vi "多点监测上位机-网络版.vi"() -> ()   [LabVIEW 2017]
uses:
  <vilib>/Utility/miscctls.llb/LVRowAndColumnTypeDef.ctl
  <vilib>/Utility/miscctls.llb/LVRowAndColumnUnsignedTypeDef.ctl
  <vilib>/Platform/TimedLoop/XDataNode/timing_clust.ctl
  <vilib>/Platform/TimedLoop/XDataNode/nitl_modes.ctl
  <vilib>/Platform/TimedLoop/XDataNode/wakeup.ctl
  <vilib>/Instr/_visa.llb/VISA Find Search Mode.ctl
  <vilib>/sound2/lvsound2.llb/Sound File Info (path).vi
  <vilib>/sound2/lvsound2.llb/Sound File Read Open.vi
  <vilib>/sound2/lvsound2.llb/Sound File Read (DBL).vi
  <vilib>/Utility/inputDevices.llb/closeMouse.vi
  <vilib>/Utility/inputDevices.llb/mouseAcquire.vi
  <vilib>/Platform/TimedLoop/XDataNode/XDataNode.xnode
  <vilib>/Platform/TimedLoop/XDataNode/XDNodeRunTimeDep.lvlib
  <vilib>/Utility/xml.llb/Read From XML File(string).vi
panel:
  out "信号-状态栏可见行数":bool=TRUE
  in  "定时器":T1
  in  "标志-定时分段?":bool=TRUE
  in  "菜单锁-报警表":bool=TRUE
  in  "菜单锁-设备表":bool=TRUE
  out "手动静音窗口VI-引用":refnum<vi>
  in  "报警列表提示索引":i32
  in  "设备列表提示索引":i32
  out "监测数量限值":cluster{"min":i32, "max":i32}
  out "监-停止信号":refnum<vi>
  in  "报警列表提示":string[](array[string])=["选行技巧：按住 ctl 可离散选择，按住 shift 可范围选择，ctl+A 选择全部行", "右键菜单：多选后 某些项可批量操作", "双击“单元格”：打开报警记录数据分析界面，可编辑结论、生成Word报表"]
  in  "设备列表提示":string[](array[string])=["选行技巧：按住 ctl 可离散选择，按住 shift 可范围选择，ctl+A 选择全部行", "右键菜单：多选后 某些项可批量操作", "双击“状态”列：启用或禁用设备（某些版本中禁用此功能）", "双击“设备信息”列：修改设备信息", "双击“一级限值”列：修改报警限值", "双击“网络地址”列：删除设备", "双击“空白行”：添加设备"]
  in  "停止信号":enum16{"内部停止信号", "外部停止信号"}(ring)
  out "新纪录通知VI":refnum<vi>
  in  "新记录簇":cluster{"新记录列表行":string[], "对应缓存文件":string}[](array[cluster])
  in  "报警记录数":i32
  in  "蜂鸣音效":waveform(dbl)[](array[waveform]) caption="数据"
  in  "新记录？":bool=TRUE
  in  "Right":i16
  in  "Left":i16
  in  "探头数":i32
  out "定时循环结构名称":string="采集探头属性"
  in  "测量状态":T2
  in  "通信单元-探头属性引用[]":refnum<vi>[](array[refnum])
  out "通信单元-改动项引用[]":refnum<vi>[](array[refnum])
  out "监测窗口VI":refnum<vi>
  out "报警记录缓存数据文件":string[](array[string])
  in  "监测模式":bool caption="方格样式"
  in  "查看报表":bool caption="方格样式"
  in  "设置":bool
  in  "通知设置":bool caption="方格样式"
  out "公司LOGO与型号":bool
  out "设备表名":string="设备列表"
  in  "串口配置":bool
  in  "设备表-修改信息":bool
  in  "设备表-报警设置":bool
  in  "状态栏-项名[]":string[](array[string])
  in  "设备表-累积定时":bool
  in  "设备表-累积清零":bool
  in  "设备表-添加设备":bool
  in  "设备表-删除设备":bool
  in  "设备排序":bool
  in  "设备表-排序":bool
  out "设备列表操作提示":string
  out "定时触发VI-引用":refnum<vi>
  out "通信单元-VI引用[]":refnum<vi>[](array[refnum])
  in  "探头属性数组":T3[](array[typedef])
  in  "菜单项-实时列表":T12=enum."禁用"
  in  "实时数据列表":i32[](listbox)
  out "报警表名":string="报警记录"
  in  "报警表-刷新":bool
  in  "报警表-预览":bool
  in  "报警表-删除":bool
  out "报警列表操作提示":string
  in  "报警表-复制":bool
  in  "菜单项-报警列表":T13=enum."预览并生成报表"
  in  "报警记录列表":i32[](listbox)
  in  "状态类型":enum16{"全部", "报警", "通信", "设置"}(ring)
  in  "暂停更新？":bool
  in  "状态栏":i32(listbox)
  in  "开机启动":bool
  in  "device ID":refnum<k1> caption="设备ID"
  in  "监测模式？":bool
  out "点到行列-实时列表":T14 caption="单元格位置"
  out "点到行列-报警记录":T14 caption="单元格位置"
  out "停止":bool=TRUE
  in  "清除状态":bool
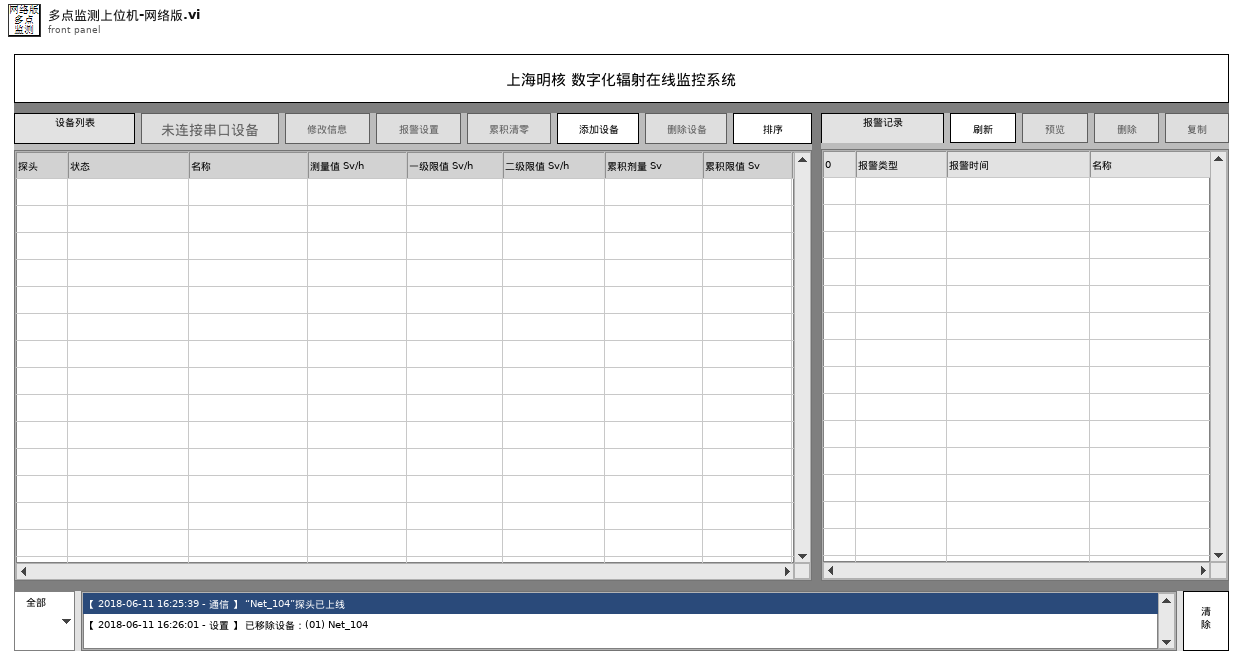
[diagram p1: front panel]
types:
  T1 = typedef "定时器枚举.ctl" = enum16{"累积定时", "导出定时"}
  T2 = typedef "测量状态.ctl" = enum16{"正常", "一级报警", "二级报警", "累积报警", "有掉线"}
  T3 = typedef "探头属性.ctl" = cluster{"探头地址与信息":T4, "测量值":T7, "限值":T8, "探头状态":T9, "累积记录":T10, "报警方式":T11}
  T4 = typedef "探测器信息.ctl" = cluster{"网络地址":string, "名称":string, "备注":string, "累积剂量":dbl, "累积限值":dbl, "硬件剂量率限值":T5, "剂量率限值1":dbl, "剂量率限值2":dbl, "报警方式":T6}
  T5 = typedef "探头剂量率限值选择.ctl" = enum16{"一级限值", "二级限值"}
  T6 = typedef "报警方式选择.ctl" = enum16{"常报警", "自动静音", "手动静音"}
  T7 = typedef "测量值.ctl" = cluster{"时间":timestamp, "数值":dbl}
  T8 = typedef "剂量率限值.ctl" = cluster{"限值1":dbl, "限值2":dbl, "探头限值":T5}
  T9 = typedef "探头状态.ctl" = enum16{"正常", "离线", "禁用", "一级报警", "二级报警", "累积报警"}
  T10 = typedef "单条累积记录.ctl" = cluster{"起始时间":timestamp, "结束时间":timestamp, "累积剂量":dbl}
  T11 = typedef "报警方式.ctl" = cluster{"报警方式":T6, "延迟计时":u16, "报警中？":bool}
  T12 = typedef "菜单项-实时列表.ctl" = enum16{"启用", "禁用", "修改探头信息", "修改报警设置", "设备排序", "重启累积时段", "累积定时", "累积清零", "添加设备", "删除设备"}
  T13 = typedef "菜单项-报警列表.ctl" = enum16{"刷新", "预览并生成报表", "删除记录", "复制选中项至剪贴板"}
  T14 = typedef "LVRowAndColumnTypeDef.ctl" = cluster{"Row":i32, "Column":i32}
  T15 = typedef "LVRowAndColumnUnsignedTypeDef.ctl" = cluster{"Row":u32, "Column":u32}
  T16 = typedef "簇-输入.ctl" = cluster{"配置文件动作":T17, "数据输入":variant}
  T17 = typedef "枚举-配置文件动作.ctl" = enum16{"初始化加载配置", "读取配置", "写入-屏幕键盘", "写入-静音延迟", "写入-主要探头类型", "写入-串口配置", "写入-累积定时", "写入-导出定时", "保存配置到文件"}
  T18 = enum32{"Invalid", "Standard", "Closed", "Hidden", "Minimized", "Maximized"}
  T19 = typedef "XDNodeRunTimeDep.lvlib/timing_clust.ctl" = cluster{"Expected End [f-1]":u64, "Actual End [f-1]":u64, "Finished Late? [f-1]":bool, "Expected End [i-1]":u64, "Actual End [i-1]":u64, "Finished Late? [i-1]":bool, "Expected Start [i]":u64, "Actual Start [i]":u64, "Expected Start [f]":u64, "Actual Start [f]":u64, "Source Name":string, "Structure Name":string, "Period":i64, "Deadline":i64, "Offset":i64, "Start":i64, "Priority":i32, "Timeout":i32, "Mode":T20, "Wakeup Reason":T21, "Error":errorcluster, "Source Type":string, "Secondary Source Type":string, "Global End Time":u64, "Global Start Time":u64, "Frame Duration":u64, "Iteration Duration":u64, "Assigned CPU":i32, "I/O Scan Engine Mode":u32}
  T20 = typedef "XDNodeRunTimeDep.lvlib/nitl_modes.ctl" = enum32{"No Change", "Process missed periods, maintain original phase", "Discard missed periods, maintain original phase", "Process missed periods, ignore original phase", "Discard missed periods, ignore original phase"}
  T21 = typedef "XDNodeRunTimeDep.lvlib/wakeup.ctl" = enum32{"Normal", "Aborted", "Asynchronous wakeup", "Timing source error", "Timed loop error", "Timeout"}
  T22 = typedef "串口配置.ctl" = cluster{"COM口":refnum<visa-resource-name>, "波特率":enum16{"9600", "19200"}, "探头地址(U8)":u8}
  T23 = typedef "串口模块输入.ctl" = cluster{"串口动作类型":T24, "串口配置":T22, "数据输入":variant}
  T24 = typedef "串口动作类型.ctl" = enum16{"读测量值", "设置报警值", "设置地址", "设置系数", "广播修改波特率", "关闭串口"}
  T25 = typedef "簇-定时配置.ctl" = cluster{"定时模式":enum16{"绝对时间", "相对时间"}, "单位":enum16{"年", "月", "日", "时", "分"}, "间隔":u8, "目标时刻":timestamp}
  T26 = typedef "改动项选择.ctl" = enum16{"未改动", "改动-启用状态", "改动-探头信息", "改动-报警限值", "动作-手动静音", "动作-重启累积时段", "动作-累积删除", "动作-重连"}
  T27 = typedef "删除记录输入.ctl" = cluster{"名称":string, "多条记录(空则全删)":T10[]}
  T28 = typedef "DB动作与数据.ctl" = cluster{"动作类型":T29, "输入数据":variant}
  T29 = typedef "DB动作类型.ctl" = enum16{"DB-文件初始化+连接", "DB-断开连接", "DB-结构初始化", "DB-加载设备", "DB-检查连接状态", "设备-登记新设备+数据表", "设备-删除设备", "设备-修改网址", "设备-修改名称+转移数据", "设备-修改备注", "设备-修改限值", "设备-累积校准", "设备-重排", "数据-获取全部", "数据-删除数据", "数据-写改累积记录+改累积剂量", "读变量-全部设备"}
  T30 = typedef "LVRectTypeDef.ctl" = cluster{"Left":i16, "Top":i16, "Right":i16, "Bottom":i16}
  T31 = typedef "Sound File Refnum.ctl" = refnum<file>
  T32 = typedef "簇-配置文件内容.ctl" = cluster{"调试模式？":bool, "屏幕键盘？":bool, "软件版本":string, "静音延迟 s":u16, "主要探头类型":T33, "串口配置":cluster{"COM口":refnum<visa-resource-name>, "波特率":enum16{"9600", "19200"}, "读写超时ms":i16, "丢包判定次数":i16}, "定时配置-累积分段":T25, "定时配置-自动导出":cluster{"定时配置-自动导出":T25, "分别导出?":bool}}
  T33 = typedef "枚举-主要探头类型.ctl" = enum16{"网络探头", "串口探头"}
  T34 = cluster{"COM口":refnum<visa-resource-name>, "波特率":enum16{"9600", "19200"}, "读写超时ms":i16, "丢包判定次数":i16}
  T35 = typedef "VISA Find Search Mode.ctl" = u32
  T36 = typedef "LVPoint32TypeDef.ctl" = cluster{"Horizontal":i32, "Vertical":i32}
  T37 = cluster{"button 1":bool, "button 2":bool, "button 3":bool, "button 4":bool}
  T38 = cluster{"Shift":bool, "Ctrl":bool, "Alt":bool, "Cmd":bool, "Opt":bool}
  T39 = typedef "eventvkey.ctl" = enum16{"ASCII", "Enter", "Return", "Shift", "Ctrl", "Alt", "Cmd", "Opt", "Caps", "NumLock", "Clear", "Break", "Up", "Down", "Left", "Right", "Insert", "Delete", "Home", "End", "PageUp", "PageDown", "Escape", "Help", "Pause", "ScrollLock", "F1", "F2", "F3", "F4", "F5", "F6", "F7", "F8", "F9", "F10", "F11", "F12", "F13", "F14", "F15", "F16", "F17", "F18", "F19", "F20", "F21", "F22", "F23", "F24", "Play", "VolumeUp", "VolumeDown", "Mute", "Two Byte Char"}
  T40 = enum8{"Enabled", "Disabled", "Disabled and Grayed Out"}
  T41 = typedef "改动项.ctl" = cluster{"改动项选择":T26, "启用？":bool, "探测器信息":T4}
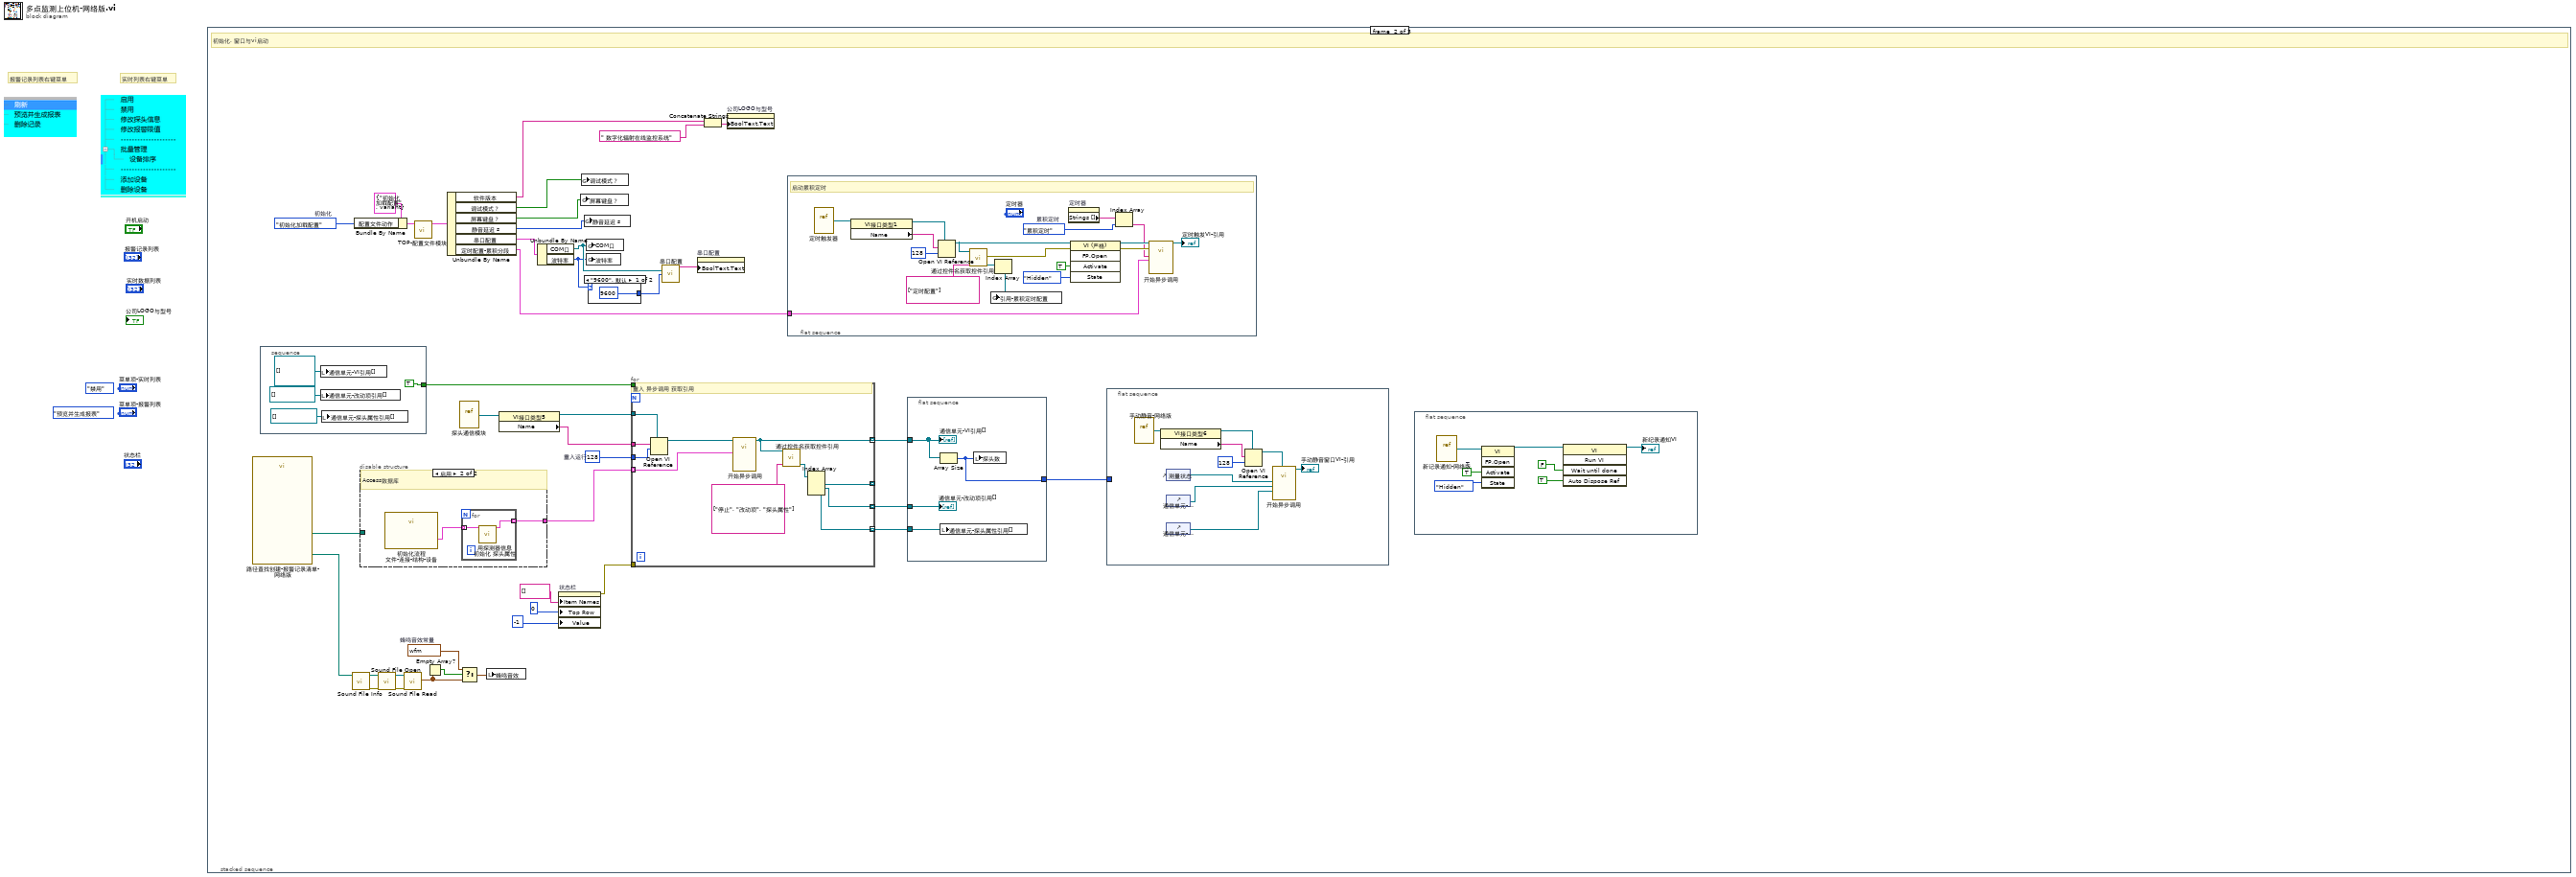
[diagram p0: block diagram]
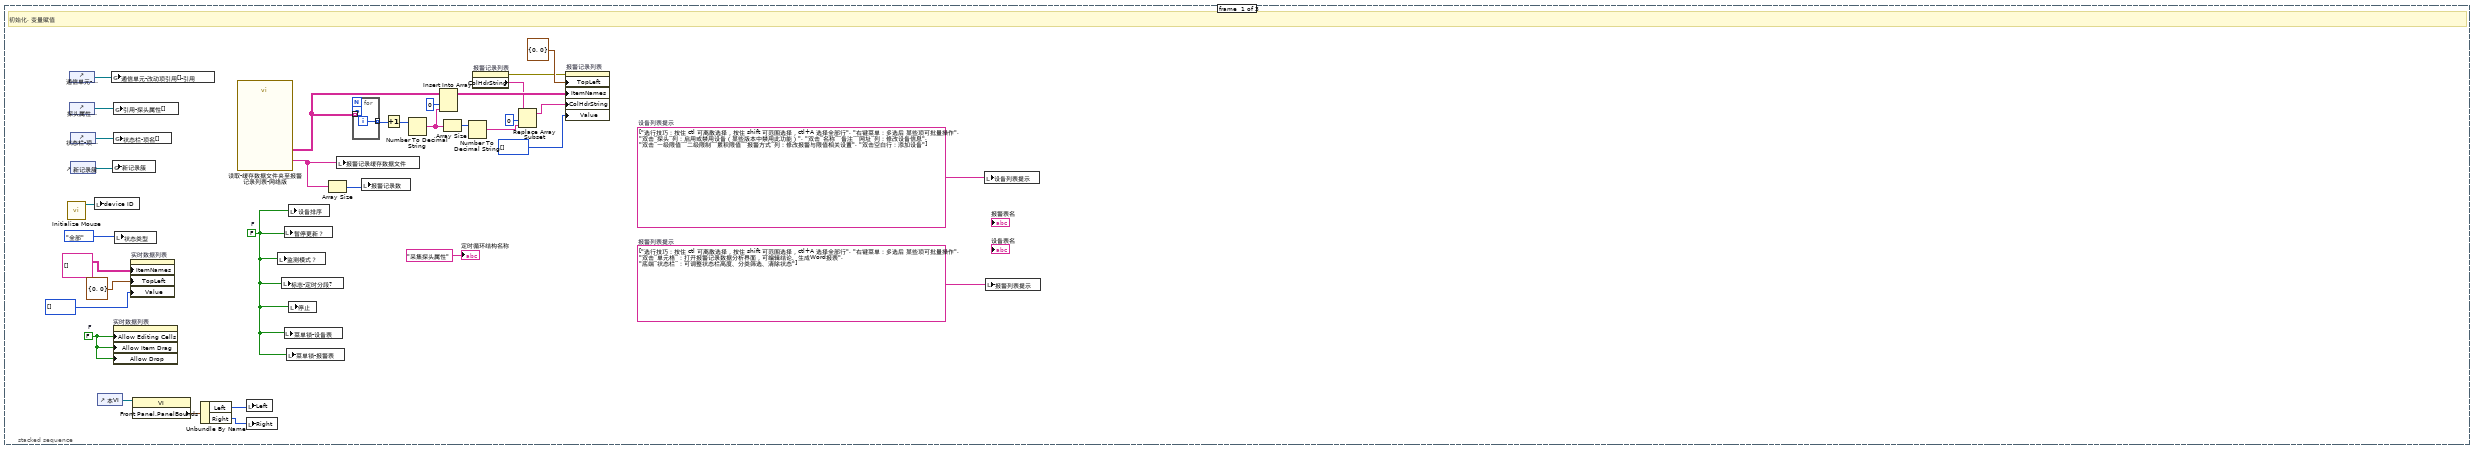
[diagram p2: hidden frame]
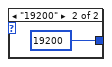
[diagram p3: hidden frame]
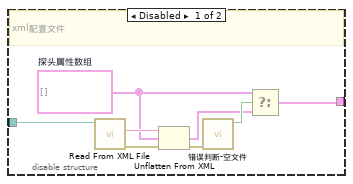
[diagram p4: hidden frame]
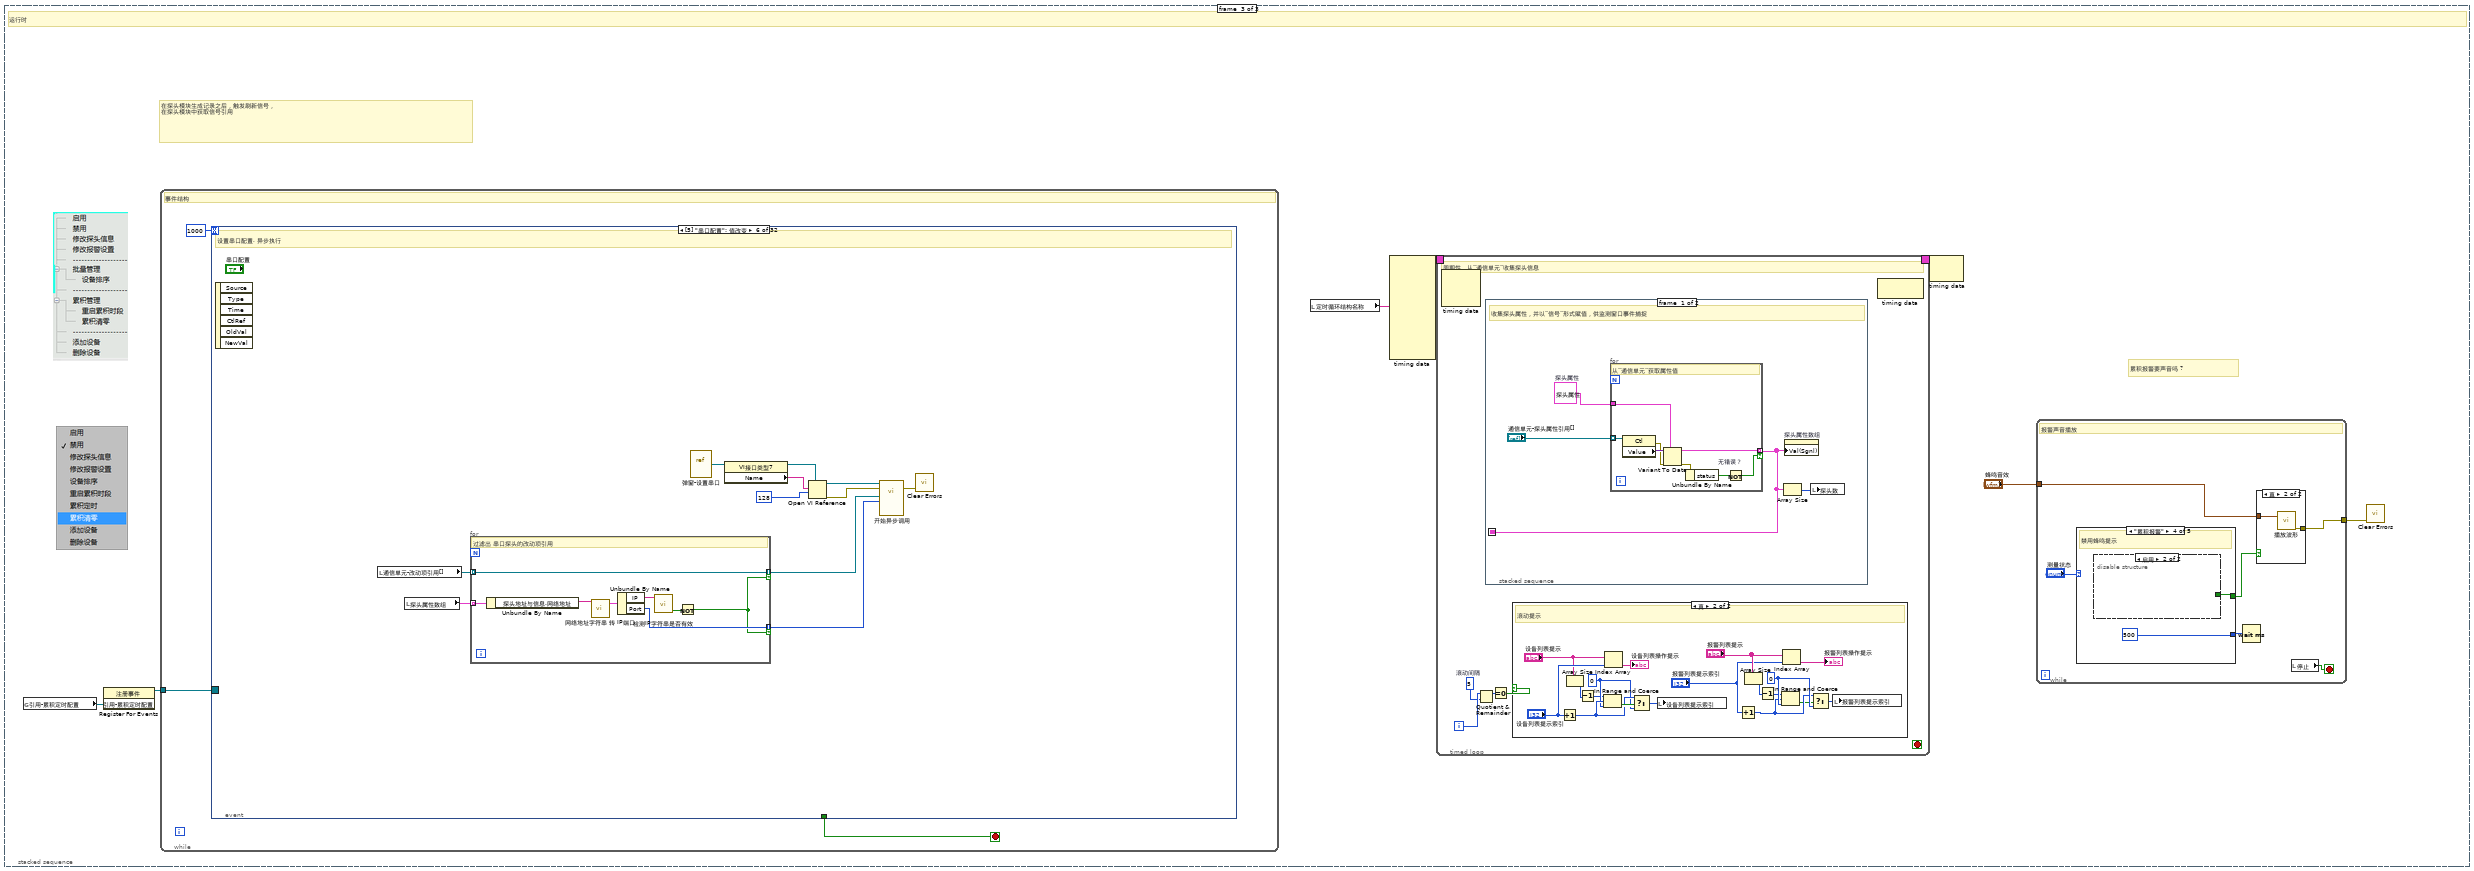
[diagram p5: hidden frame]
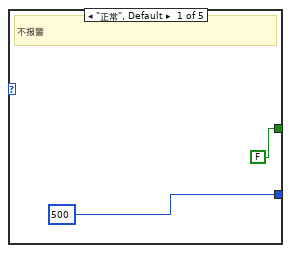
[diagram p6: hidden frame]
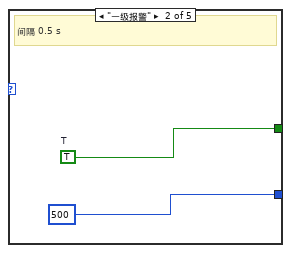
[diagram p7: hidden frame]
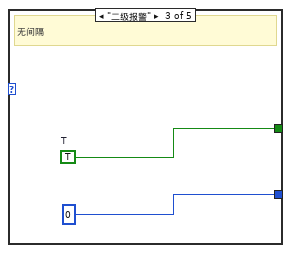
[diagram p8: hidden frame]
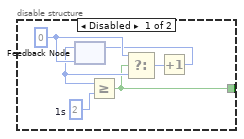
[diagram p9: hidden frame]
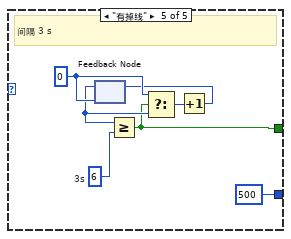
[diagram p10: hidden frame]
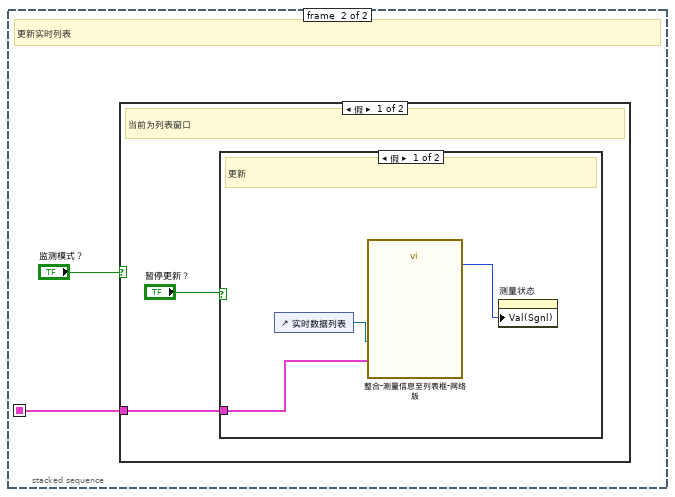
[diagram p13: hidden frame]
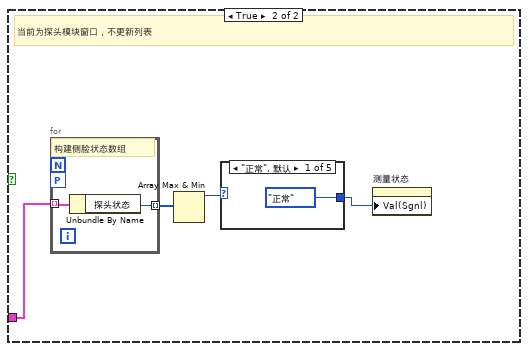
[diagram p15: hidden frame]
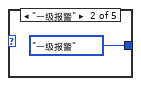
[diagram p16: hidden frame]
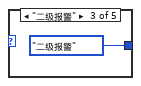
[diagram p17: hidden frame]
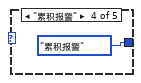
[diagram p18: hidden frame]
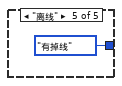
[diagram p19: hidden frame]
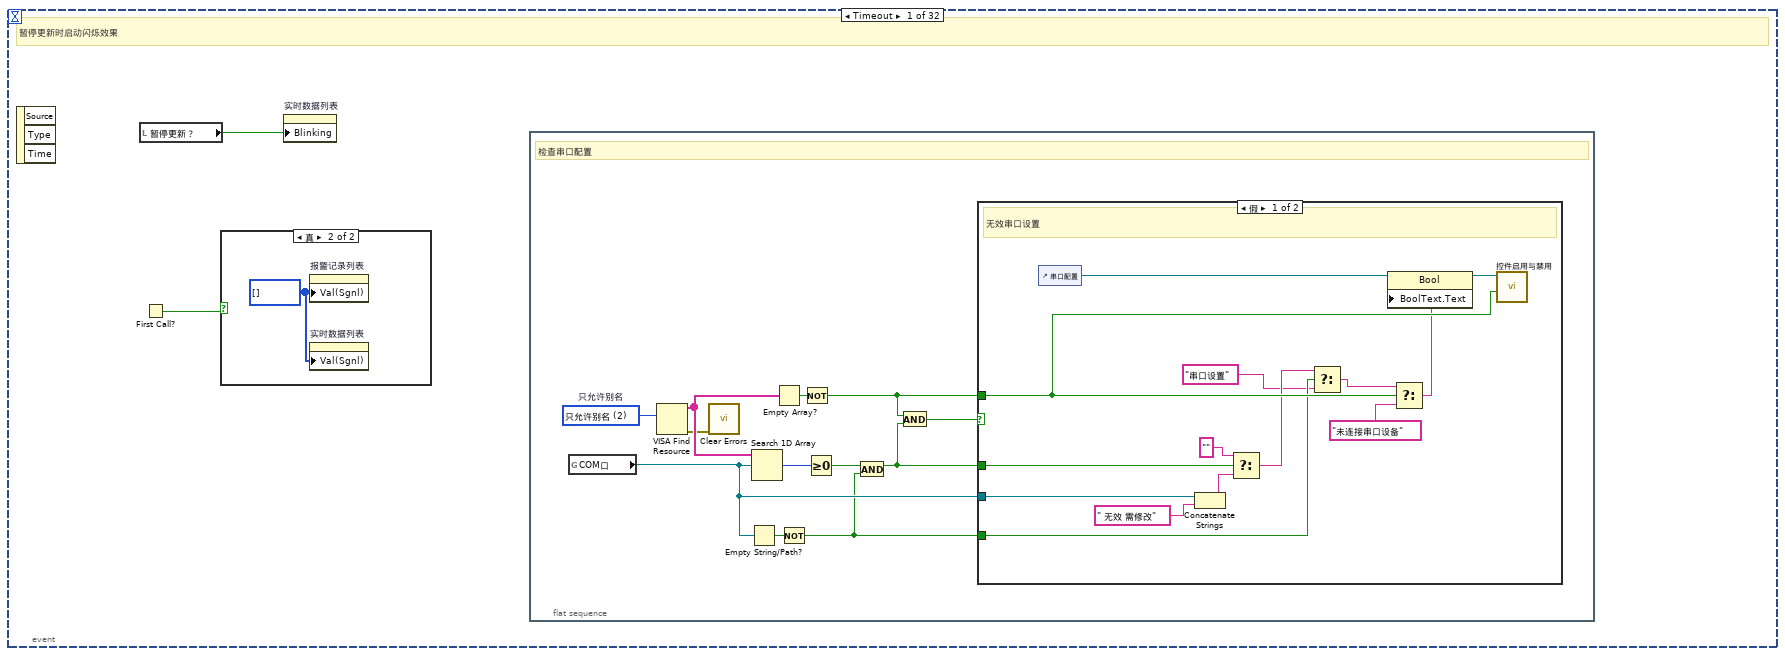
[diagram p20: hidden frame]
diagram:
  (unwired) 菜单项-报警列表."预览并生成报表" ("菜单项-报警列表")
  (unwired) 菜单项-实时列表."禁用" ("菜单项-实时列表")
  # "报警记录列表右键菜单"
  # "实时列表右键菜单"
  n1 = stacked-sequence {
    frame #0 {
      w17 = string[] ["选行技巧：按住 ctl 可离散选择，按住 shift 可范围选择，ctl+A 选择全部行", "右键菜单：多选后 某些项可批量操作", "双击“单元格”：打开报警记录数据分析界面，可编辑结论、生成Word报表", "底端“状态栏”：可调整状态栏高度、分类筛选、清除状态"]  # 报警列表提示
      w16 = string[] ["选行技巧：按住 ctl 可离散选择，按住 shift 可范围选择，ctl+A 选择全部行", "右键菜单：多选后 某些项可批量操作", "双击“探头”列：启用或禁用设备（某些版本中禁用此功能）", "双击“名称”“备注”“网址”列：修改设备信息", "双击“一级限值”“二级限制”“累积限值”“报警方式”列：修改报警与限值相关设置", "双击空白行：添加设备"]  # 设备列表提示
      w24 = FALSE  # F
      w19 = FALSE  # F
      # "初始化, 变量赋值"
      n2 = call <vilib>:"Initialize Mouse.vi"() -> ("device ID"=w33:refnum<k1>)  [unwired: 10 in, 1 out]
      n3 = control-ref of="通信单元-改动项引用[]"() -> (w15:refnum<vi>)
      n4 = control-ref of="探头属性数组"() -> (w26:refnum<vi>)
      n5 = control-ref of="状态栏-项名[]"() -> (w34:refnum<vi>)
      n6 = control-ref of="新记录簇"() -> (w27:refnum<vi>)
      n7 = local write "device ID"(w33) -> ()
      n8 = control-ref of="本VI"() -> (w32:refnum<vi>)
      n9 = global write "全局变量-35点监测.vi" "通信单元-改动项引用[]-引用"(w15) -> ()
      n10 = global write "全局变量-35点监测.vi" "新记录簇"(w27) -> ()
      n11 = property on="实时数据列表" class="多列列表框 (严格)"("Allow Editing Cells"=w19, "Allow Item Drag"=w19, "Allow Drop"=w19) -> ()  [unwired: 2 in, 2 out]
      n12 = global write "全局变量-35点监测.vi" "引用-探头属性[]"(w26) -> ()
      n13 = global write "全局变量-35点监测.vi" "状态栏-项名[]"(w34) -> ()
      n14 = local write "状态类型"(enum16{"全部", "报警", "通信", "设置"}."全部" ("状态类型")) -> ()
      n15 = property on="实时数据列表" class="MCListbox (严格)"("ItemNames"=string[][] [] ("项名"), "TopLeft"=T15 {"Row"=0, "Column"=0} ("左上可见单元格"), "Value"=i32[] [] ("报警记录列表")) -> ()  [unwired: 2 in, 2 out]
      n16 = property class="VI"(reference=w32) -> ("Front Panel.PanelBounds"=w31:T30)  [unwired: 1 in, 2 out]
      n17 = Unbundle By Name(w31) -> ("Left"=w30:i16, "Right"=w29:i16)
      n18 = call "读取-缓存数据文件夹至报警记录列表-网络版.vi"() -> ("文件名"=w28:string[], "报警记录列表"=w14:string[][])  [unwired: 8 in, 2 out]
      n19 = local write "Left"(w30) -> ()
      n20 = local write "Right"(w29) -> ()
      n21 = local write "监测模式？"(w24) -> ()
      n22 = local write "标志-定时分段?"(w24) -> ()
      n23 = local write "暂停更新？"(w24) -> ()
      n24 = local write "菜单锁-设备表"(w24) -> ()
      n25 = local write "菜单锁-报警表"(w24) -> ()
      n26 = local write "设备排序"(w24) -> ()
      n27 = local write "停止"(w24) -> ()
      n28 = Array Size(array=w28) -> (size(s)=w25:i32)
      n29 = local write "报警记录缓存数据文件"(w28) -> ()
      n30 = for {
        tunnel: w14 -> [_] mode=indexing
        tunnel: [w35] -> w13 mode=indexing
        workers-P: _ -> [_]
        i -> [w35]
      }
      n31 = local write "报警记录数"(w25) -> ()
      n32 = Increment(x=w13) -> (x+1=w10:i32[])
      n33 = Number To Decimal String(number=w10) -> (decimal integer string=w9:string[])  [unwired: 1 in]
      n34 = Insert Into Array(array=w14, index (col)=0 ("禁用的索引 (列)"), new element=w9) -> (w12:string[][])  [unwired: 1 in]
      n35 = Array Size(array=w9) -> (size(s)=w8:i32)
      n36 = Number To Decimal String(number=w8) -> (decimal integer string=w6:string)  [unwired: 1 in]
      n37 = property on="报警记录列表" class="MCListbox (严格)"() -> (error out=w3:errorcluster, "ColHdrString"=w7:string[])  [unwired: 2 in, 1 out]
      n38 = Replace Array Subset(array=w7, new element=w6, index=0 ("索引")) -> (w5:string[])
      n39 = property on="报警记录列表" class="MCListbox (严格)"(error in=w3, "TopLeft"=T15 {"Row"=0, "Column"=0} ("左上可见单元格"), "ItemNames"=w12, "ColHdrString"=w5, "Value"=i32[] [] ("报警记录列表")) -> ()  [unwired: 1 in, 2 out]
      n40 = local write "设备列表提示"(w16) -> ()
      n41 = local write "报警列表提示"(w17) -> ()
      "定时循环结构名称" <- "采集探头属性"
    }
    frame #1 {
      w38 = waveform(dbl)[] [{"t0"=timestamp(0 s since 1904-01-01), "dt"=9.070294784580499e-05, "Y"=array[2481 elements]}, {"t0"=timestamp(0 s since 1904-01-01), "dt"=9.070294784580499e-05, "Y"=array[2481 elements]}]  # 蜂鸣音效常量
      w52 = 枚举-配置文件动作."初始化加载配置"  # 初始化
      w72 = 128  # 重入运行
      # "初始化, 窗口与vi启动"
      n42 = call "路径查找创建-报警记录清单-网络版.vi"() -> ("蜂鸣音效文件路径"=w62:path, "探头属性配置文件"=w75:path)  [unwired: 2 in, 12 out]
      n43 = stacked-sequence {
        tunnel: [TRUE] -> w61
        frame #0 {
          n44 = local write "通信单元-VI引用[]"(refnum<vi>[] [] ("通信单元-VI引用[]")) -> ()
          n45 = local write "通信单元-改动项引用[]"(refnum<vi>[] [] ("通信单元-改动项引用[]")) -> ()
          n46 = local write "通信单元-探头属性引用[]"(refnum<vi>[] [] ("通信单元-探头属性引用[]")) -> ()
        }
      }
      n47 = call-poly <vilib>:"Sound File Info.vi"("path"=w62) -> ("error out"=w64:errorcluster, "path out"=w65:path)  [unwired: 7 in, 2 out]
      n48 = Bundle By Name(cluster=T16 {"配置文件动作"=enum."初始化加载配置", "数据输入"=variant} ("输入"), "配置文件动作"=w52) -> (w55:T16)
      n49 = disable-structure shown="启用" {
        disable-tunnel: w75 -> [w108 _]
        disable-tunnel: [w104 w111] -> w70
        frame Disabled {
          w103 = T3[] []  # 探头属性数组
          # "xml配置文件"
          n50 = call-poly <vilib>:"Read From XML File.vi"("XML File Path"=w108) -> ("error out"=w106:errorcluster, "XML Elements"=w105:string)  [unwired: 8 in, 1 out]
          n51 = Unflatten From XML(xml string=w105, type=w103, error in (no error)=w106) -> (value=w107:T3[], error out=w109:errorcluster)
          n52 = call "错误判断-空文件.vi"("错误输入"=w109) -> ("空文件？"=w110:bool)  [unwired: 9 in, 1 out]
          n53 = Select(t=w103, s=w110, f=w107) -> (s? t:f=w104:T3[])
        }
        frame Enabled {
          # "Access数据库"
          n54 = call "初始化流程 文件-连接-结构-设备.vi"() -> ("探测器信息[]"=w112:T4[])  [unwired: 10 in, 1 out]
          n55 = for {
            tunnel: w112 -> [w114] mode=indexing
            tunnel: [w113] -> w111 mode=indexing
            n56 = call "用探测器信息 初始化 探头属性.vi"("探测器信息"=w114) -> ("探头属性"=w113:T3)  [unwired: 10 in]
          }
        }
      }
      n57 = call-poly <vilib>:"Sound File Open.vi"("error in (no error)"=w64, "path"=w65) -> ("error out"=w63:errorcluster, "sound file refnum"=w66:T31)  [unwired: 8 in]
      n58 = call-poly <vilib>:"Sound File Read.vi"("error in (no error)"=w63, "sound file refnum"=w66) -> ("data"=w37:waveform(dbl)[])  [unwired: 5 in, 4 out]
      n59 = call "TOP-配置文件模块.vi"("输入"=w55) -> ("配置文件"=w54:T32)  [unwired: 9 in, 1 out]
      n60 = Empty Array?(array=w37) -> (empty?=w39:bool)
      n61 = Unbundle By Name(w54) -> ("软件版本"=w45:string, "调试模式？"=w49:bool, "屏幕键盘？"=w48:bool, "静音延迟 s"=w47:u16, "串口配置"=w46:T34, "定时配置-累积分段"=w50:T25)
      n62 = vi-ref "探头通信模块.vi"() -> (w74:refnum<vi>)
      n63 = Select(t=w38, s=w39, f=w37) -> (s? t:f=w36:waveform(dbl)[])
      n64 = local write "蜂鸣音效"(w36) -> ()
      n65 = property class="VI接口类型5"(reference=w74) -> (reference out=w44:refnum<vi>, "Name"=w73:string)  [unwired: 1 in, 1 out]
      n66 = Unbundle By Name(w46) -> ("COM口"=w43:refnum<visa-resource-name>, "波特率"=w41:enum16{"9600", "19200"})
      n67 = property on="状态栏" class="LstBox (严格)"("Item Names"=string[] [] ("项名"), "Top Row"=0 ("顶行"), "Value"=-1 ("状态栏")) -> (error out=w68:errorcluster)  [unwired: 2 in, 1 out]
      n68 = global write "全局变量-35点监测.vi" "屏幕键盘？"(w48) -> ()
      n69 = global write "全局变量-35点监测.vi" "调试模式？"(w49) -> ()
      n70 = global write "全局变量-35点监测.vi" "静音延迟 s"(w47) -> ()
      n71 = global write "全局变量-35点监测.vi" "COM口"(w43) -> ()
      n72 = global write "全局变量-35点监测.vi" "波特率"(w41) -> ()
      n73 = case shown="\"9600\", 默认" w41 {
        tunnel: [9600 19200] -> w40
        frame "9600", Default {
        }
        frame "19200" {
        }
      }
      n74 = for "For循环" {
        tunnel: w73 -> [w142]
        tunnel: w72 -> [w141]
        tunnel: [w137] -> w67 mode=indexing
        tunnel: [w136] -> w71 mode=indexing
        tunnel: [w135] -> w69 mode=indexing
        tunnel: w70 -> [w134] mode=indexing
        tunnel: w68 -> [_]
        tunnel: [w133] -> _ mode=indexing
        tunnel: w61 -> [_]
        tunnel: w44 -> [w132]
        # "重入 异步调用 获取引用"
        n75 = Open VI Reference(type specifier VI Refnum (for type only)=w132, vi path=w142, options=w141) -> (vi reference=w140:refnum<vi>)  [unwired: 3 in, 1 out]
        n76 = call-by-ref "开始异步调用"(reference=w140, "探头属性"=w134) -> (reference out=w137:refnum<vi>)  [unwired: 12 in, 1 out]
        n77 = call "通过控件名获取控件引用.vi"("控件名数组"=string[] ["停止", "改动项", "探头属性"], "VI引用"=w137) -> ("控件引用输出"=w139:refnum<vi>[])  [unwired: 7 in, 2 out]
        n78 = Index Array(array=w139) -> (element #1=w133:refnum<vi>, element #2=w136:refnum<vi>, element #3=w135:refnum<vi>)  [unwired: 3 in]
      }
      n79 = call "串口配置"("COM口"=w43, "波特率"=w40) -> ("Result"=w42:string)  [unwired: 12 in, 1 out]
      n80 = property on="串口配置" class="Bool"("BoolText.Text"=w42) -> ()  [unwired: 2 in, 2 out]
      n81 = Concatenate Strings(w45, " 数字化辐射在线监控系统" ("字符串")) -> (w56:string)
      n82 = property on="公司LOGO与型号" class="Bool"("BoolText.Text"=w56) -> ()  [unwired: 2 in, 2 out]
      n83 = flat-sequence {
        tunnel: w50 -> [w89]
        frame #0 {
          w80 = 定时器枚举."累积定时"  # 累积定时
          # "启动累积定时"
          n84 = vi-ref "定时触发器.vi"() -> (w93:refnum<vi>)
          n85 = property class="VI接口类型1"(reference=w93) -> (reference out=w78:refnum<vi>, "Name"=w95:string)  [unwired: 1 in, 1 out]
          n86 = Open VI Reference(type specifier VI Refnum (for type only)=w78, vi path=w95, options=128 ("选项")) -> (vi reference=w86:refnum<vi>)  [unwired: 3 in, 1 out]
          n87 = call "通过控件名获取控件引用.vi"("控件名数组"=string[] ["定时配置"], "VI引用"=w86) -> ("控件引用输出"=w91:refnum<vi>[], "错误输出"=w85:errorcluster)  [unwired: 7 in, 1 out]
          n88 = Index Array(array=w91) -> (element=w90:refnum<vi>)  [unwired: 1 in]
          n89 = global write "全局变量-35点监测.vi" "引用-累积定时配置"(w90) -> ()
          n90 = property on="定时器" class="Enum (严格)"() -> ("Strings []"=w81:string[])  [unwired: 2 in, 2 out]
          n91 = invoke class="VI (严格)" method="FP.Open"(reference=w86, error in=w85, "Activate"=TRUE ("激活？"), "State"=T18."Hidden" ("状态")) -> (reference out=w87:refnum<vi>, error out=w84:errorcluster)  [unwired: 1 in, 3 out]
          n92 = Index Array(array=w81, index=w80) -> (element=w79:string)
          n93 = call-by-ref "开始异步调用"(reference=w87, error in=w84, "定时配置"=w89, "定时器结构名"=w79) -> (reference out=→"定时触发VI-引用":refnum<vi>)  [unwired: 10 in, 1 out]
        }
      }
      n94 = flat-sequence {
        tunnel: w71 -> [w118]
        tunnel: w69 -> [w117]
        tunnel: w67 -> [w116]
        tunnel: [w115] -> w59
        frame #0 {
          n95 = Array Size(array=w116) -> (size(s)=w115:i32)
          n96 = local write "通信单元-探头属性引用[]"(w117) -> ()
          n97 = local write "探头数"(w115) -> ()
          "通信单元-VI引用[]" <- w116
          "通信单元-改动项引用[]" <- w118
        }
      }
      n98 = flat-sequence {
        tunnel: w59 -> [_]
        frame #0 {
          n99 = vi-ref "手动静音-网络版.vi"() -> (w127:refnum<vi>)
          n100 = property class="VI接口类型6"(reference=w127) -> (reference out=w119:refnum<vi>, "Name"=w125:string)  [unwired: 1 in, 1 out]
          n101 = control-ref of="测量状态"() -> (w123:refnum<vi>)
          n102 = control-ref of="通信单元-改动项引用[]"() -> (w122:refnum<vi>)
          n103 = control-ref of="通信单元-探头属性引用[]"() -> (w121:refnum<vi>)
          n104 = Open VI Reference(type specifier VI Refnum (for type only)=w119, vi path=w125, options=128 ("选项")) -> (vi reference=w124:refnum<vi>)  [unwired: 3 in, 1 out]
          n105 = call-by-ref "开始异步调用"(reference=w124, "引用-通信单元-探头属性引用[]"=w121, "引用-通信单元-改动项引用[]"=w122, "引用-测量状态"=w123) -> (reference out=→"手动静音窗口VI-引用":refnum<vi>)  [unwired: 10 in, 1 out]
        }
      }
      n106 = flat-sequence {
        frame #0 {
          w100 = TRUE  # T
          n107 = vi-ref "新记录通知-网络版.vi"() -> (w98:refnum<vi>)
          n108 = invoke class="VI" method="FP.Open"(reference=w98, "Activate"=w100, "State"=T18."Hidden" ("状态")) -> (reference out=w97:refnum<vi>)  [unwired: 2 in, 4 out]
          n109 = invoke class="VI" method="Run VI"(reference=w97, "Wait until done"=FALSE ("结束前等待"), "Auto Dispose Ref"=TRUE ("自动销毁引用")) -> (reference out=→"新纪录通知VI":refnum<vi>)  [unwired: 2 in, 4 out]
        }
      }
    }
    frame #2 {
      # "累积报警要声音吗 ?"
      # "在探头模块生成记录之后，触发刷新信号，\n在探头模块中获取信号引用"
      # "运行时"
      n110 = global read "全局变量-35点监测.vi" "引用-累积定时配置"() -> (w145:refnum<vi>)
      n111 = register-events(w145) -> (reference out=w144:refnum<event-registration>)  [unwired: 2 in, 1 out]
      n112 = while {
        tunnel: w144 -> [w237]
        stop <- w239 stop-if-true
        # "事件结构"
        n113 = event shown="[5] \"串口配置\": 值改变" {
          selector: w237 -> [_ _ w280 _ _ _ _ _ _ _ _ _ _ _ _ _ _ _ _ _ _ _ _ _ _ _ _ _ _ _ _ _]
          dyn-events: _ -> [_ _ _ _ _ _ _ _ _ _ _ _ _ _ _ _ _ _ _ _ _ _ _ _ _ _ _ _ _ _ _ _]
          timeout: 1000 -> [_ _ _ _ _ _ _ _ _ _ _ _ _ _ _ _ _ _ _ _ _ _ _ _ _ _ _ _ _ _ _ _]
          tunnel: [_ _ w281 _ _ _ _ _ _ _ _ _ _ _ _ _ _ _ _ _ _ _ _ _ _ _ _ _ _ _ _ _] -> w239
          event Timeout {
            # "暂停更新时启动闪烁效果"
            n114 = event-data() -> ()  [unwired: 1 in, 3 out]
            n115 = local read "暂停更新？"() -> (w241:bool)
            n116 = First Call?() -> (First Call?: T/F=w240:bool)
            n117 = case shown="真" w240 {
              frame False {
              }
              frame True {
                w277 = i32[] [] ("值(信号)")
                n118 = property on="报警记录列表" class="MCListbox (严格)"("Val(Sgnl)"=w277) -> ()  [unwired: 2 in, 2 out]
                n119 = property on="实时数据列表" class="MCListbox (严格)"("Val(Sgnl)"=w277) -> ()  [unwired: 2 in, 2 out]
              }
            }
            n120 = property on="实时数据列表" class="MCListbox (严格)"("Blinking"=w241) -> ()  [unwired: 2 in, 2 out]
            n121 = flat-sequence {
              frame #0 {
                w253 = T35 2 items=["仅允许规范名称"=0, "只允许别名"=2, "包含匹配别名"=3, "包含所有别名"=4]  # 只允许别名
                # "检查串口配置"
                n122 = global read "全局变量-35点监测.vi" "COM口"() -> (w245:refnum<visa-resource-name>)
                n123 = VISA Find Resource(10:w253) -> (0:w247:errorcluster, 3:w251:string[])  [unwired: 2 in, 1 out]
                n124 = call <vilib>:"Clear Errors.vi"("error in (no error)"=w247) -> ()  [unwired: 5 in, 2 out]
                n125 = Empty String/Path?(string/path=w245) -> (empty?=w244:bool)
                n126 = Search 1D Array(1D array=w251, element=w245) -> (index of element=w252:i32)  [unwired: 1 in]
                n127 = Empty Array?(array=w251) -> (empty?=w250:bool)
                n128 = Not(x=w244) -> (.not. x?=w242:bool)
                n129 = Not(x=w250) -> (.not. x?=w249:bool)
                n130 = Greater Or Equal To 0?(x=w252) -> (x >= 0?=w248:bool)
                n131 = And(x=w248, y=w242) -> (x .and. y?=w243:bool)
                n132 = And(x=w249, y=w243) -> (x .and. y?=w246:bool)
                n133 = case shown="假" w246 {
                  tunnel: w245 -> [w267 w274]
                  tunnel: w249 -> [w266 _]
                  tunnel: w243 -> [w265 _]
                  tunnel: w242 -> [w257 _]
                  frame False {
                    # "无效串口设置"
                    n134 = control-ref of="串口配置"() -> (w264:refnum<vi>)
                    n135 = Concatenate Strings(w267, " 无效 需修改") -> (w261:string)
                    n136 = Select(t="", s=w265, f=w261) -> (s? t:f=w256:string)
                    n137 = Select(t=w256, s=w257, f="串口设置") -> (s? t:f=w254:string)
                    n138 = Select(t=w254, s=w266, f="未连接串口设备") -> (s? t:f=w260:string)
                    n139 = property class="Bool"(reference=w264, "BoolText.Text"=w260) -> (reference out=w259:refnum<vi>)  [unwired: 1 in, 1 out]
                    n140 = call "控件启用与禁用.vi"("启用？"=w266, "控件引用"=w259) -> ()  [unwired: 9 in, 1 out]
                  }
                  frame True {
                    w268 = TRUE  # T
                    # "有效串口"
                    n141 = control-ref of="串口配置"() -> (w271:refnum<vi>)
                    n142 = global read "全局变量-35点监测.vi" "波特率"() -> (w272:enum16{"9600", "19200"})
                    n143 = case shown="\"9600\", 默认" w272 {
                      tunnel: [9600 19200] -> w273
                      frame "9600", Default {
                      }
                      frame "19200" {
                      }
                    }
                    n144 = call "串口配置2"("COM口"=w274, "波特率"=w273) -> ("Result"=w270:string)  [unwired: 12 in, 1 out]
                    n145 = property class="Bool"(reference=w271, "BoolText.Text"=w270) -> (reference out=w269:refnum<vi>)  [unwired: 1 in, 1 out]
                    n146 = call "控件启用与禁用.vi"("启用？"=w268, "控件引用"=w269) -> ()  [unwired: 9 in, 1 out]
                  }
                }
              }
            }
          }
          event Panel Close? {
            w279 = TRUE  # T
            # "触发停止"
            n147 = event-data() -> ()  [unwired: 1 in, 4 out]
            n148 = property on="停止信号" class="Enum (严格)"("Val(Sgnl)"=enum16{"内部停止信号", "外部停止信号"}."内部停止信号" ("值(信号)")) -> ()  [unwired: 2 in, 2 out]
            n149 = event-data("Discard?"=w279) -> ()  [unwired: 1 in, 1 out]
          }
          event "停止信号": Value Change {
            # "触发停止事件，关闭通信单元，关闭TCP连接"
            n150 = event-data() -> ("NewVal"=w282:enum16{"内部停止信号", "外部停止信号"})  [unwired: 1 in, 5 out]
            n151 = case shown="\"内部停止信号\", 默认" w282 {
              tunnel: [w283 w284] -> w281
              frame "内部停止信号", Default {
                # "内部停止，需要弹窗"
                n152 = call "显示对话框信息3"() -> ("确定"=w283:bool)  [unwired: 10 in, 1 out]
              }
              frame "外部停止信号" {
                w284 = TRUE  # T
                # "外部停止，不弹窗"
              }
            }
            "停止" <- w281
            n153 = case shown="真" w281 {
              tunnel: w280 -> [_ w285]
              frame False {
                # "取消停止"
              }
              frame True {
                # "关闭所有通信单元VI，关闭所有TCP连接，保存配置至文件"
                n154 = stacked-sequence {
                  tunnel: w285 -> [_ w288 _ _]
                  frame #0 {
                    # "保存“探头属性”和“状态栏信息”到文件，关闭鼠标引用"
                    n155 = local read "device ID"() -> (w286:refnum<k1>)
                    n156 = call-poly <vilib>:"Close Input Device.vi"("device ID"=w286) -> ()  [unwired: 9 in, 1 out]
                  }
                  frame #1 {
                    # "关闭所有通信单元VI"
                    n157 = Unregister For Events(event registration refnum=w288) -> (error out=w287:errorcluster)  [unwired: 1 in]
                    n158 = local read "定时循环结构名称"() -> (w297:string)
                    n159 = local read "通信单元-VI引用[]"() -> (w302:refnum<vi>[])
                    n160 = local read "手动静音窗口VI-引用"() -> (w294:refnum<vi>)
                    n161 = call <vilib>:"Stop Timed Structure.vi"("name"=w297) -> ()  [unwired: 10 in, 1 out]
                    n162 = local read "新纪录通知VI"() -> (w301:refnum<vi>)
                    n163 = for "For循环" {
                      tunnel: w302 -> [w306] mode=indexing
                      # "中止VI"
                      n164 = invoke class="VI (严格)" method="Abort VI"(reference=w306) -> (reference out=w303:refnum<vi>, error out=w305:errorcluster)  [unwired: 2 in, 1 out]
                      n165 = invoke class="VI (严格)" method="FP.Close"(reference=w303, error in=w305) -> (error out=w304:errorcluster)  [unwired: 1 in, 2 out]
                      n166 = call <vilib>:"Clear Errors.vi"("error in (no error)"=w304) -> ()  [unwired: 5 in, 2 out]
                    }
                    n167 = invoke class="VI (严格)" method="Abort VI"(reference=w294) -> (reference out=w295:refnum<vi>, error out=w296:errorcluster)  [unwired: 2 in, 1 out]
                    n168 = local read "定时触发VI-引用"() -> (w290:refnum<vi>)
                    n169 = invoke class="VI" method="Abort VI"(reference=w301) -> (reference out=w300:refnum<vi>, error out=w299:errorcluster)  [unwired: 2 in, 1 out]
                    n170 = invoke class="VI (严格)" method="FP.Close"(reference=w295, error in=w296) -> (error out=w293:errorcluster)  [unwired: 1 in, 2 out]
                    n171 = invoke class="VI (严格)" method="Abort VI"(reference=w290, error in=w287) -> (reference out=w292:refnum<vi>, error out=w291:errorcluster)  [unwired: 1 in, 1 out]
                    n172 = invoke class="VI" method="FP.Close"(reference=w300, error in=w299) -> (error out=w298:errorcluster)  [unwired: 1 in, 2 out]
                    n173 = call <vilib>:"Clear Errors.vi"("error in (no error)"=w298) -> ()  [unwired: 5 in, 2 out]
                    n174 = invoke class="VI (严格)" method="FP.Close"(reference=w292, error in=w291) -> (error out=w289:errorcluster)  [unwired: 1 in, 2 out]
                    n175 = call <vilib>:"Clear Errors.vi"("error in (no error)"=w293) -> ()  [unwired: 5 in, 2 out]
                    n176 = call <vilib>:"Clear Errors.vi"("error in (no error)"=w289) -> ()  [unwired: 5 in, 2 out]
                  }
                  frame #2 {
                    w312 = 串口动作类型."关闭串口"  # 关闭串口
                    # "关闭串口"
                    n177 = global read "全局变量-35点监测.vi" "COM口"() -> (w308:refnum<visa-resource-name>)
                    n178 = global read "全局变量-35点监测.vi" "波特率"() -> (w309:enum16{"9600", "19200"})
                    n179 = Bundle By Name(cluster=T22 {"COM口"="", "波特率"=enum."9600", "探头地址(U8)"=0} ("串口配置"), "COM口"=w308, "波特率"=w309) -> (w310:T22)
                    n180 = Bundle By Name(cluster=T23 {"串口动作类型"=enum."读测量值", "串口配置"={"COM口"="", "波特率"=enum."9600", "探头地址(U8)"=0}, "数据输入"=variant} ("串口模块输入"), "串口动作类型"=w312, "串口配置"=w310, "数据输入"=variant) -> (w313:T23)
                    n181 = call "TOP-串口通信模块.vi"("串口模块输入"=w313) -> ("error out"=w315:errorcluster)  [unwired: 9 in, 1 out]
                    n182 = call <vilib>:"Clear Errors.vi"("error in (no error)"=w315) -> ()  [unwired: 5 in, 2 out]
                  }
                  frame #3 {
                    # "关闭前面板"
                    n183 = control-ref of="本VI"() -> (w317:refnum<vi>)
                    n184 = invoke class="VI" method="FP.Close"(reference=w317) -> (error out=w316:errorcluster)  [unwired: 2 in, 2 out]
                    n185 = call <vilib>:"Clear Errors.vi"("error in (no error)"=w316) -> ()  [unwired: 5 in, 2 out]
                  }
                }
              }
            }
          }
          event Value Change {
            # "定时触发了,"
            n186 = event-data() -> ("NewVal"=w321:variant)  [unwired: 1 in, 5 out]
            n187 = Variant To Data(type=T25 {"定时模式"=enum."绝对时间", "单位"=enum."年", "间隔"=1, "目标时刻"=timestamp(0 s since 1904-01-01)} ("定时配置-累积分段"), Variant=w321) -> (data=w319:T25)  [unwired: 1 in, 1 out]
            n188 = Unbundle By Name(w319) -> ("目标时刻"=w318:timestamp)
            n189 = flat-sequence {
              frame #0 {
                w326 = TRUE  # T
                # "先, 设定全部重启时段的标识"
                n190 = local write "标志-定时分段?"(w326) -> ()
              }
              frame #1 {
                w327 = 菜单项-实时列表."重启累积时段"  # 重启累积
                # "再, 触发重启时段菜单操作"
                n191 = property on="菜单项-实时列表" class="Enum (严格)"("Val(Sgnl)"=w327) -> ()  [unwired: 2 in, 2 out]
              }
            }
            n192 = Format Date/Time String(time format string (%c)="%Y.%m.%d %H-%M-%S" ("时间格式字符串(%c)"), seconds (now)=w318) -> (date/time string=w323:string)  [unwired: 1 in]
            n193 = call "创建文本2"("下个_累"=w323) -> ("Result"=w322:string)  [unwired: 13 in, 1 out]
            n194 = call "状态栏-插入状态信息-35点监测专用.vi"("消息内容"=w322, "状态类型"=enum16{"全部", "报警", "通信", "设置"}."设置") -> ()  [unwired: 10 in]
          }
          event "通知设置": Value Change {
            n195 = event-data() -> ()  [unwired: 1 in, 6 out]
            n196 = vi-ref "短信通知设置.vi"() -> (w328:refnum<vi>)
            n197 = invoke class="VI" method="Run VI"(reference=w328, "Wait until done"=FALSE ("结束前等待"), "Auto Dispose Ref"=TRUE ("自动销毁引用")) -> (error out=w331:errorcluster)  [unwired: 2 in, 4 out]
            n198 = call <vilib>:"Clear Errors.vi"("error in (no error)"=w331) -> ()  [unwired: 5 in, 2 out]
          }
          event "串口配置": Value Change {
            # "设置串口配置, 异步执行"
            n199 = event-data() -> ()  [unwired: 1 in, 6 out]
            n200 = local read "通信单元-改动项引用[]"() -> (w338:refnum<vi>[])
            n201 = local read "探头属性数组"() -> (w339:T3[])
            n202 = for {
              tunnel: w339 -> [w350] mode=indexing
              tunnel: w338 -> [w346] mode=indexing
              tunnel: [w346] -> w333 mode=indexing if=w343
              tunnel: [w344] -> w332 mode=indexing if=w343
              # "过滤出 串口探头的改动项引用"
              n203 = Unbundle By Name(w350) -> ("探头地址与信息.网络地址"=w347:string)
              n204 = call "网络地址字符串 转 IP端口.vi"("IP端口字符串"=w347) -> ("IP端口"=w349:cluster{"IP":string, "Port":u16})  [unwired: 10 in]
              n205 = Unbundle By Name(w349) -> ("IP"=w348:string, "Port"=w344:u16)
              n206 = call "检测IP字符串是否有效.vi"("IP地址"=w348) -> ("有效IP？"=w345:bool)  [unwired: 10 in]
              n207 = Not(x=w345) -> (.not. x?=w343:bool)
            }
            n208 = vi-ref "弹窗-设置串口.vi"() -> (w335:refnum<vi>)
            n209 = property class="VI接口类型7"(reference=w335) -> (reference out=w334:refnum<vi>, "Name"=w342:string)  [unwired: 1 in, 1 out]
            n210 = Open VI Reference(type specifier VI Refnum (for type only)=w334, vi path=w342, options=128 ("选项")) -> (vi reference=w340:refnum<vi>, error out=w337:errorcluster)  [unwired: 3 in]
            n211 = call-by-ref "开始异步调用"(reference=w340, error in=w337, "串口探头地址"=w332, "串口通信单元-改动项引用[]"=w333) -> (error out=w336:errorcluster)  [unwired: 10 in, 1 out]
            n212 = call <vilib>:"Clear Errors.vi"("error in (no error)"=w336) -> ()  [unwired: 5 in, 2 out]
          }
          event "监测模式？": Value Change {
            n213 = event-data() -> ()  [unwired: 1 in, 6 out]
            n214 = disable-structure shown="禁用" {
              frame Disabled {
                # "没有顶层框架时候，启用“监测模式？”值改变事件"
                n215 = control-ref of="本VI"() -> (w352:refnum<vi>)
                n216 = invoke class="VI" method="FP.Open"(reference=w352, "Activate"=TRUE ("激活？"), "State"=T18."Standard" ("状态")) -> (error out=w351:errorcluster)  [unwired: 2 in, 4 out]
                n217 = call <vilib>:"Clear Errors.vi"("error in (no error)"=w351) -> ()  [unwired: 5 in, 2 out]
              }
              frame Enabled {
              }
            }
          }
          event "实时数据列表", "报警记录列表": Mouse Down {
            # "使  右击行  列表能够获取焦点"
            n218 = event-data() -> ("CtlRef"=w359:refnum<vi>, "Coords"=w361:T36)  [unwired: 1 in, 7 out]
            n219 = property class="MCListbox (严格)"(reference=w359) -> ("Label.Text"=w358:string)  [unwired: 1 in, 2 out]
            n220 = call-poly <vilib>:"Acquire Input Data.vi"("device ID"="device ID") -> ("button info"=w363:T37)  [unwired: 15 in, 3 out]
            n221 = invoke class="多列列表框 (严格)" method="Point To Row Column"(reference=w359, "Point"=w361) -> ("CellPosition"=w360:T14)  [unwired: 5 in, 6 out]
            "点到行列-实时列表" <- w360
            n222 = property on="实时数据列表" class="MCListbox (严格)"() -> ("Label.Text"=w357:string)  [unwired: 2 in, 2 out]
            n223 = Unbundle By Name "btn_2"(w363) -> ("button 2"=w362:bool)
            n224 = Equal?(x=w358, y=w357) -> (x = y?=w356:bool)
            n225 = case shown="真" w362 {
              tunnel: w359 -> [_ w379]
              tunnel: w360 -> [_ w377]
              tunnel: w356 -> [_ w367]
              frame False {
                # "不是右键"
              }
              frame True {
                w372 = TRUE  # T
                w380 = TRUE  # T
                # "右键"
                n226 = property class="多列列表框 (严格)" props=["ContentRectPosTop", "Value"](reference=w379) -> ("Value"=w376:i32[])  [unwired: 1 in, 3 out]
                n227 = Unbundle By Name(w377) -> ("Row"=w370:i32)
                n228 = Increment(x=w370) -> (x+1=w369:i32)
                n229 = Build Array(w370) -> (w378:i32[])
                n230 = Select(t="探头数", s=w367, f="报警记录数") -> (s? t:f=w365:i32)
                n231 = Less Or Equal? "点在有效信息行内？"(x=w369, y=w365) -> (x <= y?=w368:bool)
                n232 = for "For循环" {
                  tunnel: w376 -> [w397] mode=indexing
                  shift-right: [w394] -> w374
                  shift-left: w380 -> [w395]
                  tunnel: w370 -> [w392]
                  tunnel: w368 -> [w391]
                  stop <- w394 continue-if-true
                  # "在选中项之外？"
                  n233 = Not Equal?(x=w397, y=w392) -> (x != y?=w396:bool)
                  n234 = Greater Or Equal To 0?(x=w392) -> (x >= 0?=w393:bool)
                  n235 = Compound Arithmetic op=AND(w396, w395, w393, w391) -> (w394:bool)
                }
                n236 = Empty Array? "空数组？"(array=w376) -> (empty?=w375:bool)
                n237 = Select(t=w372, s=w375, f=w374) -> (s? t:f=w373:bool)
                n238 = And(x=w373, y=w368) -> (x .and. y?=w371:bool)
                n239 = case shown="真" w371 {
                  tunnel: w378 -> [_ w388]
                  tunnel: w367 -> [w381 w387]
                  tunnel: w368 -> [w382 _]
                  frame False {
                    # "在选中项之中，不赋值"
                    n240 = case shown="假" w382 {
                      tunnel: w381 -> [w383 _]
                      frame False {
                        # "点在不可选行，清空"
                        n241 = case shown="真" w383 {
                          tunnel: i32[] [] ("实时数据列表") -> [w385 w386]
                          frame False {
                            # "报警记录表"
                            n242 = property on="报警记录列表" class="MCListbox (严格)"("Val(Sgnl)"=w385) -> ()  [unwired: 2 in, 2 out]
                          }
                          frame True {
                            # "实时表"
                            n243 = property on="实时数据列表" class="MCListbox (严格)"("Val(Sgnl)"=w386) -> ()  [unwired: 2 in, 2 out]
                          }
                        }
                      }
                      frame True {
                        # "点在可选行，不赋值"
                      }
                    }
                  }
                  frame True {
                    # "在选中项之外，赋值"
                    n244 = case shown="真" w387 {
                      tunnel: w388 -> [w389 w390]
                      frame False {
                        n245 = property on="报警记录列表" class="MCListbox (严格)"("Val(Sgnl)"=w389) -> ()  [unwired: 2 in, 2 out]
                      }
                      frame True {
                        n246 = property on="实时数据列表" class="MCListbox (严格)"("Val(Sgnl)"=w390) -> ()  [unwired: 2 in, 2 out]
                      }
                    }
                  }
                }
              }
            }
          }
          event "监测模式": Value Change {
            # "被顶层框架引用的，触发值改变事件。"
            # "切换到 方格 样式 界面"
            n247 = event-data() -> ()  [unwired: 1 in, 6 out]
            n248 = local read "探头数"() -> (w401:i32)
            n249 = local read "暂停更新？"() -> (w404:bool)
            n250 = Equal To 0?(x=w401) -> (x = 0?=w402:bool)
            n251 = Or(x=w402, y=w404) -> (x .or. y?=w403:bool)
            n252 = Less Or Equal?(x=w401, y=32) -> (x <= y?=w399:bool)
            n253 = local write "监测模式"(FALSE ("监测模式")) -> ()
            n254 = case shown="真" w399 {
              tunnel: w403 -> [_ w406]
              tunnel: w401 -> [_ w405]
              frame False {
                # "超过32个探头，不能打开监测界面"
                n255 = call "显示对话框信息4"() -> ()  [unwired: 10 in, 2 out]
              }
              frame True {
                # "32个探头内可打开监测界面"
                n256 = case shown="假" w406 {
                  tunnel: w405 -> [w408 _]
                  frame False {
                    # "正常更新列表中，表示没有未完成的设置操作"
                    n257 = case shown="0..2, 默认" w408 {
                      tunnel: [w434 w436 w438 w440 w442 w444 w446 w448 w450 w452] -> w410
                      tunnel: [cluster{"min":i32, "max":i32} {"min"=0, "max"=2} ("监测数量限值") cluster{"min":i32, "max":i32} {"min"=3, "max"=4} ("监测数量限值") cluster{"min":i32, "max":i32} {"min"=5, "max"=6} ("监测数量限值") cluster{"min":i32, "max":i32} {"min"=7, "max"=8} ("监测数量限值") cluster{"min":i32, "max":i32} {"min"=9, "max"=12} ("监测数量限值") cluster{"min":i32, "max":i32} {"min"=13, "max"=16} ("监测数量限值") cluster{"min":i32, "max":i32} {"min"=17, "max"=20} ("监测数量限值") cluster{"min":i32, "max":i32} {"min"=21, "max"=24} ("监测数量限值") cluster{"min":i32, "max":i32} {"min"=25, "max"=28} ("监测数量限值") cluster{"min":i32, "max":i32} {"min"=29, "max"=32} ("监测数量限值")] -> w407
                      frame 0..2, Default {
                        n258 = vi-ref "探头窗口-2-网络版.vi"() -> (w434:refnum<vi>)
                      }
                      frame 3, 4 {
                        n259 = vi-ref "探头窗口-4-网络版.vi"() -> (w436:refnum<vi>)
                      }
                      frame 5, 6 {
                        n260 = vi-ref "探头窗口-6-网络版.vi"() -> (w438:refnum<vi>)
                      }
                      frame 7, 8 {
                        n261 = vi-ref "探头窗口-8-网络版.vi"() -> (w440:refnum<vi>)
                      }
                      frame 9..12 {
                        n262 = vi-ref "探头窗口-12-网络版.vi"() -> (w442:refnum<vi>)
                      }
                      frame 13..16 {
                        n263 = vi-ref "探头窗口-16-网络版.vi"() -> (w444:refnum<vi>)
                      }
                      frame 17..20 {
                        n264 = vi-ref "探头窗口-20-网络版.vi"() -> (w446:refnum<vi>)
                      }
                      frame 21..24 {
                        n265 = vi-ref "探头窗口-24-4列-网络版.vi"() -> (w448:refnum<vi>)
                      }
                      frame 25..28 {
                        n266 = vi-ref "探头窗口-28-4列-网络版.vi"() -> (w450:refnum<vi>)
                      }
                      frame 29..32 {
                        n267 = vi-ref "探头窗口-32-4列-网络版.vi"() -> (w452:refnum<vi>)
                      }
                    }
                    "监测数量限值" <- w407
                    n268 = invoke on="运行VI" class="VI" method="Run VI"(reference=w410, "Wait until done"=FALSE ("结束前等待"), "Auto Dispose Ref"=TRUE ("自动销毁引用")) -> (reference out=w415:refnum<vi>, error out=w416:errorcluster)  [unwired: 2 in, 3 out]
                    n269 = control-ref of="本VI"() -> (w412:refnum<vi>)
                    n270 = disable-structure shown="启用" {
                      disable-tunnel: w416 -> [w430 w431]
                      disable-tunnel: w415 -> [w429 w432]
                      disable-tunnel: w412 -> [w428 _]
                      disable-tunnel: [w425 w431] -> w411
                      disable-tunnel: [w424 w432] -> w409
                      frame Disabled {
                        n271 = invoke on="打开前面板" class="VI" method="FP.Open"(reference=w429, error in=w430, "Activate"=TRUE ("激活？"), "State"=T18."Maximized" ("状态")) -> (reference out=w424:refnum<vi>, error out=w427:errorcluster)  [unwired: 1 in, 3 out]
                        n272 = property class="VI"(reference=w428, error in=w427, "FP.State"=T18."Hidden" ("前面板窗口:状态")) -> (error out=w425:errorcluster)  [unwired: 1 out]
                      }
                      frame Enabled {
                      }
                    }
                    n273 = call <vilib>:"Clear Errors.vi"("error in (no error)"=w411) -> ()  [unwired: 5 in, 2 out]
                    n274 = stacked-sequence {
                      tunnel: w409 -> [w419 _]
                      frame #0 {
                        # "获取外部停止命令"
                        n275 = call "通过控件名获取控件引用.vi"("控件名数组"=string[] ["外部停止命令？"], "VI引用"=w419) -> ("控件引用输出"=w420:refnum<vi>[])  [unwired: 7 in, 2 out]
                        n276 = Index Array(array=w420) -> (element=→"监-停止信号":refnum<vi>)  [unwired: 1 in]
                        "监测窗口VI" <- w419
                      }
                      frame #1 {
                        # "模式切换"
                        n277 = property on="监测模式？" class="Bool (严格)"("Val(Sgnl)"=TRUE ("更新列表？")) -> ()  [unwired: 2 in, 2 out]
                      }
                    }
                  }
                  frame True {
                    # "存在未完成的设置操作，弹窗提示"
                    n278 = call "显示对话框信息2"() -> ()  [unwired: 10 in, 2 out]
                  }
                }
              }
            }
          }
          event "查看报表": Value Change {
            # "打开文件路径"
            n279 = event-data() -> ()  [unwired: 1 in, 6 out]
            n280 = call "路径查找创建-报警记录清单-网络版.vi"() -> ("导出记录"=w454:path, "报表文件夹"=w455:path)  [unwired: 2 in, 12 out]
            n281 = call "cmd打开文件夹.vi"("文件路径"=w455) -> ("error out"=w453:errorcluster)  [unwired: 10 in]
            n282 = call "cmd打开文件夹.vi"("error in (no error)"=w453, "文件路径"=w454) -> ()  [unwired: 9 in, 1 out]
          }
          event "状态栏-项名[]": Value Change {
            # "在其他VI里改变值，在此处处理"
            n283 = event-data() -> ()  [unwired: 1 in, 6 out]
            n284 = local read "状态类型"() -> (w461:enum16{"全部", "报警", "通信", "设置"})
            n285 = Array Size(array="状态栏-项名[]") -> (size(s)=w464:i32)
            n286 = Decrement(x=w464) -> (x-1=w465:i32)
            n287 = Index Array "获取新增项"(array="状态栏-项名[]", index=w465) -> (element=w460:string)
            n288 = Equal To 0?(x=w461) -> (x = 0?=w462:bool)
            n289 = case shown="假" w462 {
              tunnel: w461 -> [w482 _]
              tunnel: w460 -> [w480 _]
              tunnel: [w477 w483] -> w458
              frame False {
                # "按关键词过滤"
                n290 = property on="状态类型" class="Enum (严格)"() -> ("Strings []"=w476:string[])  [unwired: 2 in, 2 out]
                n291 = Index Array "当前关键词"(array=w476, index=w482) -> (element=w479:string)
                n292 = Match Pattern(string=w480, regular expression=w479, offset (0)=20 ("偏移量(0)")) -> (offset past match=w478:i32)  [unwired: 3 out]
                n293 = Greater Or Equal To 0?(x=w478) -> (x >= 0?=w477:bool)
              }
              frame True {
                w483 = TRUE  # T
                # "显示全部"
              }
            }
            n294 = control-ref of="状态栏"() -> (w459:refnum<vi>)
            n295 = case shown="真" w458 {
              tunnel: w459 -> [_ w475]
              tunnel: w460 -> [_ w471]
              tunnel: [_ w466] -> w456
              frame False {
                # "未匹配，不添加"
              }
              frame True {
                # "添加，并置为左上可见"
                n296 = call-poly "多态-列表插入项名.vi"("项名"=w471, "限定行数(500)"=u32 500, "LstBox引用句柄"=w475) -> ("引用输出"=w474:refnum<vi>)  [unwired: 8 in]
                n297 = property class="LstBox"(reference=w474) -> (reference out=w473:refnum<vi>, error out=w472:errorcluster, "Item Names"=w470:string[])  [unwired: 1 in]
                n298 = Array Size(array=w470) -> (size(s)=w469:i32)
                n299 = Decrement(x=w469) -> (x-1=w468:i32)
                n300 = property class="LstBox"(reference=w473, error in=w472, "Top Row"=w468) -> (error out=w466:errorcluster)  [unwired: 1 out]
              }
            }
            n301 = property on="信号-状态栏可见行数" class="Bool (严格)"(error in=w456, "Val(Sgnl)"=FALSE ("值(信号)")) -> ()  [unwired: 1 in, 2 out]
          }
          event Pane Size {
            # "窗口11 是状态栏所在窗格, 大小变化, 触发可见状态信息量调整事件"
            n302 = event-data() -> ()  [unwired: 1 in, 6 out]
            n303 = Wait (ms)(milliseconds to wait=u32 10 ("等待时间（毫秒）")) -> ()  [unwired: 1 out]
            n304 = property on="信号-状态栏可见行数" class="Bool (严格)"("Val(Sgnl)"=FALSE ("值(信号)")) -> ()  [unwired: 2 in, 2 out]
          }
          event "信号-状态栏可见行数": Value Change {
            # "状态栏更新值, 或状态栏窗口大小变化, 尽量多的显示状态信息"
            n305 = event-data() -> ()  [unwired: 1 in, 6 out]
            n306 = control-ref of="状态栏"() -> (w486:refnum<vi>)
            n307 = while {
              shift-right: [w509] -> _
              shift-left: w486 -> [w496]
              stop <- w487 stop-if-true
              w489 = TRUE  # T
              # "多行的单元格, 强制拉回一格, 并认为已是最右"
              # "调整直到显示行足够多且到底"
              n308 = property class="LstBox (严格)"(reference=w496) -> (reference out=w499:refnum<vi>, "Item Names"=w502:string[], "Number of Rows"=w501:u32)  [unwired: 1 in, 1 out]
              n309 = Array Size(array=w502) -> (size(s)=w494:i32)
              n310 = Decrement(x=w501) -> (x-1=w497:u32)
              n311 = Subtract(x=w494, y=w497) -> (x-y=w492:u32)
              n312 = Less Or Equal?(x=w494, y=w497) -> (x <= y?=w500:bool)
              n313 = Decrement(x=w494) -> (x-1=w493:i32)
              n314 = In Range and Coerce(upper limit=w493, x=w492, lower limit=u32 0 ("下限")) -> (coerced(x)=w491:u32, In Range?=w490:bool)
              n315 = case shown="假" w500 {
                tunnel: w499 -> [w511 w515]
                tunnel: [w510 w513] -> w498
                tunnel: w491 -> [w512 _]
                frame False {
                  # "项数>行数, 则重新设置"
                  n316 = property class="LstBox (严格)"(reference=w511, "Top Row"=w512) -> (reference out=w510:refnum<vi>)  [unwired: 1 in, 1 out]
                }
                frame True {
                  # "项数<=行数, 则0置顶"
                  n317 = property class="LstBox (严格)"(reference=w515, "Top Row"=0 ("顶行")) -> (reference out=w513:refnum<vi>)  [unwired: 1 in, 1 out]
                }
              }
              n318 = property class="LstBox (严格)"(reference=w498) -> (reference out=w509:refnum<vi>, "Item Names"=w508:string[], "Top Row"=w507:i32, "Number of Rows"=w506:u32)  [unwired: 1 in, 1 out]
              n319 = Decrement(x=w506) -> (x-1=w503:u32)
              n320 = Array Size(array=w508) -> (size(s)=w505:i32)
              n321 = Add(x=w507, y=w503) -> (x+y=w504:u32)
              n322 = Less Or Equal?(x=w505, y=w504) -> (x <= y?=w488:bool)
              n323 = Select(t=w488, s=w490, f=w489) -> (s? t:f=w487:bool)
            }
          }
          event "状态类型": Value Change {
            n324 = event-data() -> ()  [unwired: 1 in, 6 out]
            n325 = local read "状态栏-项名[]"() -> (w523:string[])
            n326 = Equal To 0?(x="状态类型") -> (x = 0?=w525:bool)
            n327 = case shown="假" w525 {
              tunnel: "状态类型" -> [w533 _]
              tunnel: w523 -> [w532 w545]
              tunnel: [w530 w545] -> w517
              frame False {
                # "按关键词过滤"
                n328 = property on="状态类型" class="Enum (严格)"() -> ("Strings []"=w529:string[])  [unwired: 2 in, 2 out]
                n329 = Index Array "当前关键词"(array=w529, index=w533) -> (element=w528:string)
                n330 = Concatenate Strings(w528, " 】 ") -> (w526:string)
                n331 = for "For循环" {
                  tunnel: w532 -> [w535] mode=indexing
                  tunnel: w526 -> [w538]
                  shift-right: [w534] -> w530
                  shift-left: string[] [] ("项名") -> [w536]
                  # "过滤关键词"
                  n332 = Match Pattern(string=w535, regular expression=w538, offset (0)=20 ("偏移量(0)")) -> (offset past match=w540:i32)  [unwired: 3 out]
                  n333 = Greater Or Equal To 0?(x=w540) -> (x >= 0?=w537:bool)
                  n334 = case shown="真" w537 {
                    tunnel: w536 -> [w541 w544]
                    tunnel: w535 -> [_ w543]
                    tunnel: [w541 w542] -> w534
                    frame False {
                      # "不匹配"
                    }
                    frame True {
                      # "匹配"
                      n335 = Insert Into Array(array=w544, new element=w543) -> (w542:string[])  [unwired: 1 in]
                    }
                  }
                }
              }
              frame True {
                # "显示全部"
              }
            }
            n336 = Array Size(array=w517) -> (size(s)=w518:i32)
            n337 = Decrement(x=w518) -> (x-1=w520:i32)
            n338 = control-ref of="状态栏"() -> (w516:refnum<vi>)
            n339 = Less Than 0?(x=w520) -> (x < 0?=w519:bool)
            n340 = Select(t=0, s=w519, f=w520) -> (s? t:f=w522:i32)
            n341 = property class="LstBox (严格)"(reference=w516, "Item Names"=w517, "Top Row"=w522) -> ()  [unwired: 1 in, 2 out]
          }
          event "清除状态": Value Change {
            n342 = event-data() -> ()  [unwired: 1 in, 6 out]
            n343 = control-ref of="状态栏"() -> (w550:refnum<vi>)
            n344 = property class="LstBox (严格)"(reference=w550, "Item Names"=string[] [] ("项名")) -> ()  [unwired: 1 in, 2 out]
            n345 = local read "状态栏-项名[]"() -> (w548:string[])
            n346 = local read "状态类型"() -> (w546:enum16{"全部", "报警", "通信", "设置"})
            n347 = Equal To 0?(x=w546) -> (x = 0?=w549:bool)
            n348 = case shown="假" w549 {
              tunnel: w546 -> [w557 _]
              tunnel: w548 -> [w556 _]
              tunnel: [w553 string[] [] ("项名")] -> w547
              frame False {
                # "关键词以外的，保留"
                n349 = property on="状态类型" class="Enum (严格)"() -> ("Strings []"=w552:string[])  [unwired: 2 in, 2 out]
                n350 = Index Array "当前关键词"(array=w552, index=w557) -> (element=w555:string)
                n351 = for "For循环" {
                  tunnel: w556 -> [w559] mode=indexing
                  tunnel: w555 -> [w562]
                  shift-right: [w558] -> w553
                  shift-left: string[] [] ("项名") -> [w560]
                  # "过滤关键词"
                  n352 = Match Pattern(string=w559, regular expression=w562, offset (0)=20 ("偏移量(0)")) -> (offset past match=w564:i32)  [unwired: 3 out]
                  n353 = Less Than 0? "不匹配？"(x=w564) -> (x < 0?=w561:bool)
                  n354 = case shown="假" w561 {
                    tunnel: w560 -> [w565 w568]
                    tunnel: w559 -> [_ w567]
                    tunnel: [w565 w566] -> w558
                    frame False {
                      # "匹配\n不保留"
                    }
                    frame True {
                      # "不匹配\n保留"
                      n355 = Insert Into Array(array=w568, new element=w567) -> (w566:string[])  [unwired: 1 in]
                    }
                  }
                }
              }
              frame True {
                # "全部清除"
              }
            }
            n356 = local write "状态栏-项名[]"(w547) -> ()
          }
          event "实时数据列表": Double Click {
            w585 = enum16{"正常", "离线", "禁用", "一级报警", "二级报警"}."离线"  # 探头状态-在线
            w587 = enum16{"正常", "离线", "禁用", "一级报警", "二级报警"}."禁用"  # 探头状态-禁用
            # "使 双击 可寻找到对应的列，并触发菜单处理事件，使打开修改弹窗"
            n357 = event-data() -> ("CtlRef"=w589:refnum<vi>, "Coords"=w593:T36, "PlatMods"=w573:T38)  [unwired: 1 in, 6 out]
            n358 = property class="MCListbox (严格)"(reference=w589) -> ("Value"=w591:i32[])  [unwired: 1 in, 2 out]
            n359 = invoke class="多列列表框 (严格)" method="Point To Row Column"(reference=w589, "Point"=w593) -> ("CellPosition"=w594:T14)  [unwired: 5 in, 6 out]
            n360 = Unbundle By Name(w573) -> ("Shift"=w575:bool, "Ctrl"=w574:bool)
            n361 = Not Or(1:w574, 2:w575) -> (0:w571:bool)
            n362 = Unbundle By Name(w594) -> ("Row"=w579:i32, "Column"=w592:i32)
            n363 = Index Array(array=w591) -> (element=w590:i32)  [unwired: 1 in]
            n364 = Index Array(array="探头属性数组", index=w590) -> (element=w588:T3)
            n365 = Array Size(array="探头属性数组") -> (size(s)=w582:i32)
            n366 = Unbundle By Name(w588) -> ("探头状态"=w584:T9)
            n367 = Decrement(x=w582) -> (x-1=w570:i32)
            n368 = In Range and Coerce(upper limit=w570, x=w579, lower limit=0 ("下限")) -> (In Range?=w580:bool)  [unwired: 1 out]
            n369 = Not Equal? "启用？"(x=w584, y=w587) -> (x != y?=w586:bool)
            n370 = Not Equal? "在线？"(x=w585, y=w584) -> (x != y?=w583:bool)
            n371 = And(x=w580, y=w571) -> (x .and. y?=w572:bool)
            n372 = case shown="假" w572 {
              tunnel: w589 -> [_ w607]
              tunnel: w592 -> [_ w606]
              tunnel: w586 -> [_ w605]
              tunnel: w583 -> [_ w604]
              tunnel: w579 -> [w599 _]
              tunnel: [w596 w603] -> w578
              tunnel: [w597 w602] -> w577
              frame False {
                # "无效行"
                n373 = Greater Than 0?(x=w599) -> (x > 0?=w598:bool)
                n374 = case shown="真" w598 {
                  tunnel: [_ w600] -> w597
                  tunnel: [_ w601] -> w596
                  frame False {
                    # "标题行，不执行"
                  }
                  frame True {
                    w601 = 菜单项-实时列表."添加设备"  # 添加设备
                    # "空白行，添加设备"
                    n375 = global read "全局变量-35点监测.vi" "调试模式？"() -> (w600:bool)
                  }
                }
              }
              frame True {
                # "有效行，范围内"
                n376 = case shown="0" w606 {
                  tunnel: [u16 0 ("修改探头信息") w614 w615 w617] -> w603
                  tunnel: w607 -> [_ _ _ _]
                  tunnel: w605 -> [_ w612 _ w619]
                  tunnel: [w609 w613 w616 w618] -> w602
                  tunnel: w604 -> [_ _ _ w620]
                  frame -1, Default {
                    w609 = FALSE  # F
                    # "不触发"
                  }
                  frame 0 {
                    w610 = 菜单项-实时列表."启用"  # 启用
                    w611 = 菜单项-实时列表."禁用"  # 禁用
                    w613 = FALSE  # f
                    # "禁用此双击动作, 用处不大"
                    # "序号列，禁用或启用探头"
                    n377 = Select(t=w611, s=w612, f=w610) -> (s? t:f=w614:T12)
                  }
                  frame 2, 9, 10 {
                    w615 = 菜单项-实时列表."修改探头信息"  # 修改探头信息
                    w616 = TRUE  # T
                    # "探头信息列，修改探头信息"
                  }
                  frame 4, 5, 7, 8 {
                    w617 = 菜单项-实时列表."修改报警设置"  # 修改限值
                    # "一级、二级、累积限值、报警方式 列"
                    n378 = disable-structure shown="启用" {
                      disable-tunnel: w620 -> [w623 _]
                      disable-tunnel: w619 -> [w622 _]
                      disable-tunnel: [w621 w624] -> w618
                      frame Disabled {
                        # "好像没有必要"
                        n379 = And(x=w623, y=w622) -> (x .and. y?=w621:bool)
                      }
                      frame Enabled {
                        w624 = TRUE  # T
                        # "无条件执行"
                      }
                    }
                  }
                }
              }
            }
            n380 = case shown="真" w577 {
              tunnel: w578 -> [_ w595]
              frame False {
              }
              frame True {
                # "是否触发"
                n381 = property on="菜单项-实时列表" class="Enum (严格)"("Val(Sgnl)"=w595) -> ()  [unwired: 2 in, 2 out]
              }
            }
          }
          event "报警记录列表": Double Click {
            # "历史数据列表双击，删除记录提示"
            n382 = event-data() -> ("CtlRef"=w632:refnum<vi>, "Coords"=w639:T36, "PlatMods"=w637:T38)  [unwired: 1 in, 6 out]
            n383 = invoke class="多列列表框 (严格)" method="Point To Row Column"(reference=w632, "Point"=w639) -> ("CellPosition"=w640:T14)  [unwired: 5 in, 6 out]
            "点到行列-报警记录" <- w640
            n384 = property class="MCListbox (严格)"(reference=w632) -> ("ItemNames"=w631:string[][])  [unwired: 1 in, 2 out]
            n385 = Unbundle By Name(w637) -> ("Shift"=w636:bool, "Ctrl"=w635:bool)
            n386 = Not Or "或非"(1:w635, 2:w636) -> (0:w633:bool)
            n387 = Array Size(array=w631) -> (size(s)=w629:i32[])
            n388 = Unbundle By Name(w640) -> ("Row"=w627:i32)  [unwired: 1 out]
            n389 = Index Array(array=w629) -> (element=w628:i32)  [unwired: 1 in]
            n390 = Decrement(x=w628) -> (x-1=w625:i32)
            n391 = Greater Or Equal? "有效行？"(x=w625, y=w627) -> (x >= y?=w626:bool)
            n392 = Greater Or Equal To 0? "非标题？"(x=w627) -> (x >= 0?=w638:bool)
            n393 = And(x=w626, y=w638) -> (x .and. y?=w630:bool)
            n394 = And(x=w630, y=w633) -> (x .and. y?=w634:bool)
            n395 = case shown="真" w634 {
              frame False {
                # "无效行"
              }
              frame True {
                # "有效行"
                n396 = property on="菜单项-报警列表" class="Enum (严格)"("Val(Sgnl)"=enum16{"刷新", "预览并生成报表", "删除记录"}."预览并生成报表" ("菜单项-报警列表")) -> ()  [unwired: 2 in, 2 out]
              }
            }
          }
          event "实时数据列表": Value Change {
            # "控制菜单按钮启用状态"
            n397 = event-data() -> ("NewVal"=w642:i32[])  [unwired: 1 in, 5 out]
            n398 = case shown="假" "菜单锁-设备表" {
              tunnel: w642 -> [w645 _]
              frame False {
                w653 = TRUE  # T
                # "在没有进行菜单操作时"
                n399 = Array Size(array=w645) -> (size(s)=w644:i32)
                n400 = case shown="0" w644 {
                  tunnel: w653 -> [w661 w662 w663]
                  tunnel: [w661 w662 w663] -> w652
                  tunnel: [w661 w662 w663] -> w651
                  tunnel: [w661 w662 _] -> w650
                  tunnel: [_ w662 _] -> w649
                  tunnel: [_ w662 w663] -> w648
                  tunnel: [_ w662 w663] -> w647
                  tunnel: [_ w662 w663] -> w646
                  frame 0 {
                    # "没有选中"
                  }
                  frame 1 {
                    # "单选"
                  }
                  frame 2, Default {
                    # "多选"
                  }
                }
                n401 = control-ref of="设备表-报警设置"() -> (w659:refnum<vi>)
                n402 = control-ref of="设备表-累积定时"() -> (w658:refnum<vi>)
                n403 = control-ref of="设备表-修改信息"() -> (w660:refnum<vi>)
                n404 = control-ref of="设备表-累积清零"() -> (w657:refnum<vi>)
                n405 = control-ref of="设备表-添加设备"() -> (w656:refnum<vi>)
                n406 = control-ref of="设备表-排序"() -> (w654:refnum<vi>)
                n407 = control-ref of="设备表-删除设备"() -> (w655:refnum<vi>)
                n408 = call "控件启用与禁用.vi"("启用？"=w648, "控件引用"=w659) -> ()  [unwired: 9 in, 1 out]
                n409 = call "控件启用与禁用.vi"("启用？"=w646, "控件引用"=w655) -> ()  [unwired: 9 in, 1 out]
                n410 = call "控件启用与禁用.vi"("启用？"=w649, "控件引用"=w660) -> ()  [unwired: 9 in, 1 out]
                n411 = call "控件启用与禁用.vi"("启用？"=w652, "控件引用"=w654) -> ()  [unwired: 9 in, 1 out]
                n412 = call "控件启用与禁用.vi"("启用？"=w651, "控件引用"=w656) -> ()  [unwired: 9 in, 1 out]
                n413 = call "控件启用与禁用.vi"("启用？"=w647, "控件引用"=w657) -> ()  [unwired: 9 in, 1 out]
                n414 = call "控件启用与禁用.vi"("启用？"=w650, "控件引用"=w658) -> ()  [unwired: 9 in, 1 out]
              }
              frame True {
                # "正在进行菜单操作, 或者需要保持状态时"
              }
            }
          }
          event "报警记录列表": Value Change {
            # "控制菜单按钮启用状态"
            n415 = event-data() -> ("NewVal"=w665:i32[])  [unwired: 1 in, 5 out]
            n416 = case shown="假" "菜单锁-报警表" {
              tunnel: w665 -> [w676 _]
              frame False {
                w674 = TRUE  # T
                # "为在菜单操作中, 未锁定, 可以执行"
                n417 = Array Size(array=w676) -> (size(s)=w675:i32)
                n418 = case shown="2, 默认" w675 {
                  tunnel: w674 -> [w677 w678 w679]
                  tunnel: [w677 w678 w679] -> w667
                  tunnel: [_ w678 _] -> w669
                  tunnel: [_ w678 w679] -> w668
                  tunnel: [_ w678 w679] -> w666
                  frame 0 {
                    # "没选中"
                  }
                  frame 1 {
                    # "单选"
                  }
                  frame 2, Default {
                    # "多选"
                  }
                }
                n419 = control-ref of="报警表-刷新"() -> (w670:refnum<vi>)
                n420 = control-ref of="报警表-预览"() -> (w671:refnum<vi>)
                n421 = control-ref of="报警表-复制"() -> (w673:refnum<vi>)
                n422 = control-ref of="报警表-删除"() -> (w672:refnum<vi>)
                n423 = call "控件启用与禁用.vi"("启用？"=w667, "控件引用"=w670) -> ()  [unwired: 9 in, 1 out]
                n424 = call "控件启用与禁用.vi"("启用？"=w669, "控件引用"=w671) -> ()  [unwired: 9 in, 1 out]
                n425 = call "控件启用与禁用.vi"("启用？"=w668, "控件引用"=w672) -> ()  [unwired: 9 in, 1 out]
                n426 = call "控件启用与禁用.vi"("启用？"=w666, "控件引用"=w673) -> ()  [unwired: 9 in, 1 out]
              }
              frame True {
                # "锁定了, 不可执行"
              }
            }
          }
          event "实时数据列表": Key Down {
            # "实时表 快捷键操作"
            n427 = event-data() -> ("VKey"=w681:T39, "PlatMods"=w680:T38)  [unwired: 1 in, 8 out]
            n428 = case shown="\"Delete\"" w681 {
              tunnel: w680 -> [_ _]
              frame Default {
              }
              frame "Delete" {
                # "删除设备"
                n429 = property on="设备表-删除设备" class="Bool"() -> ("DisabledEnum"=w682:T40)  [unwired: 2 in, 2 out]
                n430 = case shown="默认" w682 {
                  frame "Enabled" {
                    # "确定当前可操作"
                    n431 = property on="菜单项-实时列表" class="Enum (严格)"("Val(Sgnl)"=菜单项-实时列表."删除设备" ("值(信号)")) -> ()  [unwired: 2 in, 2 out]
                  }
                  frame Default {
                    # "当前不可操作"
                  }
                }
              }
            }
          }
          event "报警记录列表": Key Down {
            # "快捷键操作"
            n432 = event-data() -> ("VKey"=w684:T39)  [unwired: 1 in, 9 out]
            n433 = case shown="\"Enter\", \"Return\"" w684 {
              frame "ASCII", Default {
              }
              frame "Enter", "Return" {
                # "打开记录"
                n434 = property on="报警表-预览" class="Bool"() -> ("DisabledEnum"=w685:T40)  [unwired: 2 in, 2 out]
                n435 = case shown="\"Enabled\"" w685 {
                  frame "Enabled" {
                    # "可执行操作"
                    n436 = property on="菜单项-报警列表" class="Enum (严格)"("Val(Sgnl)"=菜单项-报警列表."预览并生成报表" ("菜单项-报警列表")) -> ()  [unwired: 2 in, 2 out]
                  }
                  frame "Disabled", Default {
                    # "不可执行"
                  }
                }
              }
              frame "Delete" {
                # "删除记录操作"
                n437 = property on="报警表-删除" class="Bool"() -> ("DisabledEnum"=w687:T40)  [unwired: 2 in, 2 out]
                n438 = case shown="\"Enabled\"" w687 {
                  frame "Enabled" {
                    # "可执行"
                    n439 = property on="菜单项-报警列表" class="Enum (严格)"("Val(Sgnl)"=菜单项-报警列表."删除记录" ("菜单项-报警列表")) -> ()  [unwired: 2 in, 2 out]
                  }
                  frame "Disabled", Default {
                    # "不可执行"
                  }
                }
              }
            }
          }
          event "设备表-添加设备", "设备表-报警设置", "设备表-修改信息", "设备表-删除设备", "设备表-累积清零", "设备表-排序", "设备表-累积定时", "报警表-刷新", "报警表-预览", "报警表-删除", "报警表-复制": Value Change {
            w706 = enum16{"刷新", "预览并生成报表", "删除记录", "复制选中项至剪贴板"}."刷新" ("值(信号)")
            w714 = 菜单项-实时列表."修改探头信息" ("值(信号)")
            # "排序功能由其他按钮实现, 此处无用"
            # "菜单项按钮"
            n440 = event-data() -> ("CtlRef"=w734:refnum<vi>)  [unwired: 1 in, 5 out]
            n441 = control-ref of="设备表-修改信息"() -> (w741:refnum<vi>)
            n442 = control-ref of="设备表-报警设置"() -> (w740:refnum<vi>)
            n443 = control-ref of="设备表-累积定时"() -> (w739:refnum<vi>)
            n444 = control-ref of="设备表-累积清零"() -> (w738:refnum<vi>)
            n445 = control-ref of="设备表-添加设备"() -> (w737:refnum<vi>)
            n446 = control-ref of="设备表-删除设备"() -> (w736:refnum<vi>)
            n447 = control-ref of="设备表-排序"() -> (w735:refnum<vi>)
            n448 = Equal?(x=w734, y=w739) -> (x = y?=w719:bool)
            n449 = Equal?(x=w734, y=w735) -> (x = y?=w715:bool)
            n450 = Equal?(x=w734, y=w738) -> (x = y?=w718:bool)
            n451 = Equal?(x=w734, y=w737) -> (x = y?=w717:bool)
            n452 = Equal?(x=w734, y=w740) -> (x = y?=w725:bool)
            n453 = Equal?(x=w734, y=w741) -> (x = y?=w727:bool)
            n454 = Equal?(x=w734, y=w736) -> (x = y?=w716:bool)
            n455 = Compound Arithmetic op=OR ("复合运算")(w727, w725, w719, w718, w717, w716, w715) -> (w729:bool)
            n456 = local read "菜单锁-设备表"() -> (w694:bool)
            n457 = Select(t=w714, s=w727, f=w714) -> (s? t:f=w713:T12)
            n458 = Not(x=w694) -> (.not. x?=w692:bool)
            n459 = Select(t=菜单项-实时列表."修改报警设置" ("值(信号)"), s=w725, f=w713) -> (s? t:f=w712:T12)
            n460 = Select(t=菜单项-实时列表."累积定时" ("值(信号)"), s=w719, f=w712) -> (s? t:f=w711:T12)
            n461 = Select(t=菜单项-实时列表."累积清零" ("值(信号)"), s=w718, f=w711) -> (s? t:f=w710:T12)
            n462 = Select(t=菜单项-实时列表."添加设备" ("值(信号)"), s=w717, f=w710) -> (s? t:f=w709:T12)
            n463 = Select(t=菜单项-实时列表."删除设备" ("值(信号)"), s=w716, f=w709) -> (s? t:f=w708:T12)
            n464 = Select(t=菜单项-实时列表."设备排序" ("值(信号)"), s=w715, f=w708) -> (s? t:f=w707:T12)
            n465 = And(x=w729, y=w692) -> (x .and. y?=w693:bool)
            n466 = case shown="真" w693 {
              tunnel: w707 -> [_ w742]
              frame False {
                # "没操作"
              }
              frame True {
                # "有操作"
                n467 = property on="菜单项-实时列表" class="Enum (严格)"("Val(Sgnl)"=w742) -> ()  [unwired: 2 in, 2 out]
              }
            }
            n468 = control-ref of="报警表-刷新"() -> (w733:refnum<vi>)
            n469 = control-ref of="报警表-预览"() -> (w732:refnum<vi>)
            n470 = control-ref of="报警表-复制"() -> (w730:refnum<vi>)
            n471 = control-ref of="报警表-删除"() -> (w731:refnum<vi>)
            n472 = Equal?(x=w734, y=w733) -> (x = y?=w702:bool)
            n473 = Equal?(x=w734, y=w730) -> (x = y?=w699:bool)
            n474 = Equal?(x=w734, y=w732) -> (x = y?=w701:bool)
            n475 = Equal?(x=w734, y=w731) -> (x = y?=w700:bool)
            n476 = Compound Arithmetic op=OR ("复合运算")(w702, w701, w700, w699) -> (w728:bool)
            n477 = Select(t=w706, s=w702, f=w706) -> (s? t:f=w698:enum16{"刷新", "预览并生成报表", "删除记录", "复制选中项至剪贴板"})
            n478 = Select(t=enum16{"刷新", "预览并生成报表", "删除记录", "复制选中项至剪贴板"}."预览并生成报表" ("值(信号)"), s=w701, f=w698) -> (s? t:f=w697:enum16{"刷新", "预览并生成报表", "删除记录", "复制选中项至剪贴板"})
            n479 = Select(t=enum16{"刷新", "预览并生成报表", "删除记录", "复制选中项至剪贴板"}."删除记录" ("值(信号)"), s=w700, f=w697) -> (s? t:f=w696:enum16{"刷新", "预览并生成报表", "删除记录", "复制选中项至剪贴板"})
            n480 = Select(t=enum16{"刷新", "预览并生成报表", "删除记录", "复制选中项至剪贴板"}."复制选中项至剪贴板" ("值(信号)"), s=w699, f=w696) -> (s? t:f=w695:enum16{"刷新", "预览并生成报表", "删除记录", "复制选中项至剪贴板"})
            n481 = local read "菜单锁-报警表"() -> (w690:bool)
            n482 = Not(x=w690) -> (.not. x?=w689:bool)
            n483 = And(x=w728, y=w689) -> (x .and. y?=w691:bool)
            n484 = case shown="真" w691 {
              tunnel: w695 -> [_ w743]
              frame False {
                # "没操作"
              }
              frame True {
                # "有操作"
                n485 = property on="菜单项-报警列表" class="Enum (严格)"("Val(Sgnl)"=w743) -> ()  [unwired: 2 in, 2 out]
              }
            }
          }
          event "实时数据列表": Shortcut Menu Activation? {
            w746 = FALSE  # F
            w749 = "修改探头信息" ("项名称")
            w757 = "修改报警设置" ("项名称")
            w767 = "禁用" ("项名称")
            w766 = "启用" ("项名称")
            # "排序改由单独按钮实现"
            # "探头信息 即使离线情况下也能修改"
            # "配置菜单项-实时列表"
            n486 = event-data() -> ("CtlRef"=w760:refnum<vi>, "MenuRef"=w759:refnum<k9>)  [unwired: 1 in, 5 out]
            n487 = property class="多列列表框 (严格)"(reference=w760) -> ("Value"=w770:i32[])  [unwired: 1 in, 2 out]
            n488 = Array Size(array=w770) -> (size(s)=w768:i32)
            n489 = Equal?(x=w768, y=1) -> (x = y?=w748:bool)
            n490 = disable-structure shown="启用" {
              disable-tunnel: w770 -> [w775 _]
              disable-tunnel: [w774 _] -> w765
              disable-tunnel: [w773 _] -> w764
              disable-tunnel: [w772 _] -> w755
              disable-tunnel: w748 -> [w771 _]
              frame Disabled {
                n491 = case shown="真" w771 {
                  tunnel: [w776 w778] -> w773
                  tunnel: [w776 w787] -> w774
                  tunnel: w775 -> [_ w786]
                  tunnel: [w776 w777] -> w772
                  frame False {
                    w776 = TRUE  # T
                    # "多选"
                  }
                  frame True {
                    # "单项选择，根据启用状态动态修改菜单项"
                    n492 = local read "探头属性数组"() -> (w784:T3[])
                    n493 = Index Array(array=w786) -> (element=w785:i32)  [unwired: 1 in]
                    n494 = Index Array(array=w784, index=w785) -> (element=w783:T3)
                    n495 = Unbundle By Name(w783) -> ("探头状态"=w781:T9)
                    n496 = Not Equal?(x=探头状态."离线" ("探头状态"), y=w781) -> (x != y?=w779:bool)
                    n497 = Not Equal?(x=w781, y=探头状态."禁用" ("探头状态")) -> (x != y?=w778:bool)
                    n498 = Not(x=w778) -> (.not. x?=w787:bool)
                    n499 = And "连接？"(x=w779, y=w778) -> (x .and. y?=w777:bool)
                  }
                }
              }
              frame Enabled {
              }
            }
            n500 = Set Menu Item Info(7:w766, 9:w765, 10:w766, 11:w759) -> (0:w762:errorcluster, 3:w763:refnum<k9>)  [unwired: 3 in]
            n501 = Set Menu Item Info(7:w767, 8:w762, 9:w764, 10:w767, 11:w763) -> (0:w752:errorcluster, 3:w753:refnum<k9>)  [unwired: 2 in]
            n502 = disable-structure shown="启用" {
              disable-tunnel: [w788 w789] -> w756
              disable-tunnel: w755 -> [w788 _]
              frame Disabled {
              }
              frame Enabled {
                w789 = TRUE  # T
              }
            }
            n503 = Set Menu Item Info(7:w757, 8:w752, 9:w756, 10:w757, 11:w753) -> (0:w751:errorcluster, 3:w750:refnum<k9>)  [unwired: 2 in]
            n504 = Set Menu Item Info(7:w749, 8:w751, 9:w748, 10:w749, 11:w750) -> (0:w747:errorcluster, 3:w745:refnum<k9>)  [unwired: 2 in]
            n505 = Set Menu Item Info(7:"设备排序" ("项名称"), 8:w747, 9:w746, 11:w745) -> ()  [unwired: 3 in, 2 out]
            n506 = local read "暂停更新？"() -> (w754:bool)
            n507 = Empty Array?(array=w770) -> (empty?=w769:bool)
            n508 = Or(x=w769, y=w754) -> (x .or. y?=w758:bool)
            n509 = event-data("Discard?"=w758) -> ()  [unwired: 1 in, 1 out]
          }
          event "报警记录列表": Shortcut Menu Activation? {
            w791 = "预览并生成报表" ("项标识符")
            # "菜单项启用状态，仅单选可 ”打开报表预览“ 项"
            n510 = event-data() -> ("CtlRef"=w799:refnum<vi>, "MenuRef"=w795:refnum<k9>)  [unwired: 1 in, 5 out]
            n511 = property class="多列列表框 (严格)"(reference=w799) -> ("Value"=w794:i32[])  [unwired: 1 in, 2 out]
            n512 = Array Size(array=w794) -> (size(s)=w793:i32)
            n513 = Equal? "单项？"(x=w793, y=1) -> (x = y?=w790:bool)
            n514 = Set Menu Item Info(7:w791, 9:w790, 10:w791, 11:w795) -> ()  [unwired: 3 in, 2 out]
            n515 = local read "暂停更新？"() -> (w796:bool)
            n516 = Empty Array?(array=w794) -> (empty?=w798:bool)
            n517 = Or(x=w798, y=w796) -> (x .or. y?=w797:bool)
            n518 = event-data("Discard?"=w797) -> ()  [unwired: 1 in, 1 out]
          }
          event "实时数据列表": Shortcut Menu Selection (User) {
            # "实时列表-菜单选择"
            n519 = event-data() -> ("ItemTag"=w802:string)  [unwired: 1 in, 7 out]
            n520 = property on="菜单项-实时列表" class="Enum (严格)"() -> ("Strings []"=w801:string[])  [unwired: 2 in, 2 out]
            n521 = for "For循环" {
              tunnel: w801 -> [w806] mode=indexing
              tunnel: w802 -> [w805]
              tunnel: [w803] -> w800
              i -> [w803]
              stop <- w804 stop-if-true
              # "寻找匹配项"
              n522 = Equal?(x=w806, y=w805) -> (x = y?=w804:bool)
            }
            n523 = property on="菜单项-实时列表" class="Enum (严格)"("Val(Sgnl)"=w800) -> ()  [unwired: 2 in, 2 out]
          }
          event "报警记录列表": Shortcut Menu Selection (User) {
            # "处理报警列表菜单事件"
            n524 = event-data() -> ("ItemTag"=w809:string)  [unwired: 1 in, 7 out]
            n525 = property on="菜单项-报警列表" class="Enum (严格)"() -> ("Strings []"=w808:string[])  [unwired: 2 in, 2 out]
            n526 = for "For循环" {
              tunnel: w808 -> [w813] mode=indexing
              tunnel: w809 -> [w812]
              tunnel: [w810] -> w807
              i -> [w810]
              stop <- w811 stop-if-true
              # "寻找匹配项"
              n527 = Equal?(x=w813, y=w812) -> (x = y?=w811:bool)
            }
            n528 = property on="菜单项-报警列表" class="Enum (严格)"("Val(Sgnl)"=w807) -> ()  [unwired: 2 in, 2 out]
          }
          event Value Change {
            # "实时列表，菜单事件处理"
            n529 = event-data() -> ("CtlRef"=w819:refnum<vi>, "NewVal"=w816:T12)  [unwired: 1 in, 4 out]
            n530 = flat-sequence {
              tunnel: [w821] -> w815
              frame #0 {
                w821 = TRUE  # T
                n531 = local write "菜单锁-设备表"(w821) -> ()
              }
            }
            n532 = local read "点到行列-实时列表"() -> (w818:T14)
            n533 = local read "暂停更新？"() -> (w817:bool)
            n534 = case shown="假" w817 {
              tunnel: w819 -> [_ _]
              tunnel: w818 -> [w828 _]
              tunnel: w816 -> [w824 _]
              tunnel: w815 -> [w823 _]
              tunnel: [w823 _] -> w814
              frame False {
                w826 = T41 {"改动项选择"=enum."未改动", "启用？"=FALSE, "探测器信息"={"网络地址"="", "名称"="", "备注"="", "累积剂量"=0.0, "累积限值"=0.0, "硬件剂量率限值"=enum."一级限值", "剂量率限值1"=0.0, "剂量率限值2"=0.0, "报警方式"=enum."常报警"}}  # 改动项
                # "非暂停发送状态，可以产生菜单事件"
                n535 = local read "通信单元-改动项引用[]"() -> (w827:refnum<vi>[])
                n536 = local read "探头属性数组"() -> (w822:T3[])
                n537 = local read "实时数据列表"() -> (w825:i32[])
                n538 = case shown="\"修改探头信息\"" w824 {
                  tunnel: w825 -> [w833 w855 w894 w932 _ w970 w1010 _ w1080 _]
                  tunnel: w822 -> [w832 w854 w895 w930 _ w971 w1009 _ w1079 _]
                  tunnel: w828 -> [_ _ _ _ _ _ _ _ _ _]
                  tunnel: w826 -> [w835 w857 w902 w929 _ w973 w1006 _ _ _]
                  tunnel: w827 -> [w834 w856 w901 w931 _ w974 w1008 _ _ _]
                  frame "启用" {
                    # "启用探头"
                    n539 = for "For循环" {
                      tunnel: w833 -> [w845] mode=indexing
                      tunnel: w834 -> [w852]
                      tunnel: w835 -> [w849]
                      tunnel: w832 -> [w847]
                      shift-right: [w837] -> w829
                      shift-left: "" -> [w836]
                      w851 = TRUE  # T
                      # "按列表选中项索引，修改"
                      n540 = Index Array(array=w847, index=w845) -> (element=w846:T3)
                      n541 = Index Array(array=w852, index=w845) -> (element=w850:refnum<vi>)
                      n542 = Unbundle By Name(w846) -> ("探头地址与信息.名称"=w843:string)
                      n543 = Increment(x=w845) -> (x+1=w844:i32)
                      n544 = call "状态信息-启用"("探头号"=w844, "探头信息"=w843) -> ("Result"=w838:string)  [unwired: 12 in, 1 out]
                      n545 = Bundle By Name(cluster=w849, "改动项选择"=改动项选择."改动-启用状态" ("改动项"), "启用？"=w851) -> (w848:T41)
                      n546 = property class="Ctl"(reference=w850, "Value"=w848) -> ()  [unwired: 1 in, 2 out]
                      n547 = Concatenate Strings("L-----------------------------------" ("字符串"), w838, "\r") -> (w839:string)
                      n548 = Concatenate Strings(w836, w839) -> (w837:string)
                    }
                    n549 = call "状态栏-插入状态信息-35点监测专用.vi"("消息内容"=w829, "状态类型"=enum16{"全部", "报警", "通信", "设置"}."设置") -> ()  [unwired: 10 in]
                  }
                  frame "禁用" {
                    # "禁用探头"
                    n550 = call "显示对话框信息5"() -> ("确定"=w853:bool)  [unwired: 10 in, 1 out]
                    n551 = case shown="真" w853 {
                      tunnel: w857 -> [_ w864]
                      tunnel: w856 -> [_ w863]
                      tunnel: w855 -> [_ w862]
                      tunnel: w854 -> [_ w861]
                      frame False {
                      }
                      frame True {
                        n552 = for "For循环" {
                          tunnel: w862 -> [w875] mode=indexing
                          tunnel: w863 -> [w882]
                          tunnel: w864 -> [w879]
                          tunnel: w861 -> [w877]
                          shift-right: [w865] -> w858
                          shift-left: "" -> [w867]
                          w881 = FALSE  # F
                          # "按列表选中项索引，修改"
                          n553 = Index Array(array=w877, index=w875) -> (element=w876:T3)
                          n554 = Index Array(array=w882, index=w875) -> (element=w880:refnum<vi>)
                          n555 = Unbundle By Name(w876) -> ("探头地址与信息.名称"=w873:string)
                          n556 = Increment(x=w875) -> (x+1=w874:i32)
                          n557 = call "状态信息-禁用"("探头号"=w874, "探头信息"=w873) -> ("Result"=w868:string)  [unwired: 12 in, 1 out]
                          n558 = Bundle By Name(cluster=w879, "改动项选择"=改动项选择."改动-启用状态" ("改动项"), "启用？"=w881) -> (w878:T41)
                          n559 = property class="Ctl"(reference=w880, "Value"=w878) -> (error out=w872:errorcluster)  [unwired: 1 in, 1 out]
                          n560 = Concatenate Strings("L-----------------------------------" ("字符串"), w868, "\r") -> (w866:string)
                          n561 = Concatenate Strings(w867, w866) -> (w865:string)
                          n562 = call <vilib>:"Clear Errors.vi"("error in (no error)"=w872) -> ()  [unwired: 5 in, 2 out]
                        }
                        n563 = call "状态栏-插入状态信息-35点监测专用.vi"("消息内容"=w858, "状态类型"=enum16{"全部", "报警", "通信", "设置"}."设置") -> ()  [unwired: 10 in]
                      }
                    }
                  }
                  frame "修改探头信息" {
                    w884 = enum16{"新建设备", "编辑设备"}."编辑设备"  # 编辑
                    # "防止命名冲突 , 每次只能改一个探头的名称"
                    n564 = global read "全局变量-35点监测.vi" "屏幕键盘？"() -> (w897:bool)
                    n565 = Index Array(array=w894) -> (element=w890:i32)  [unwired: 1 in]
                    n566 = case shown="真" w897 {
                      tunnel: [_ w927] -> w887
                      frame False {
                      }
                      frame True {
                        # "打开软键盘"
                        n567 = call "cmd启动屏幕键盘.vi"("软键盘开关"=enum16{"关闭", "打开"}."打开") -> ("error out"=w927:errorcluster)  [unwired: 9 in, 1 out]
                      }
                    }
                    n568 = Increment(x=w890) -> (x+1=w891:i32)
                    n569 = Index Array(array=w895, index=w890) -> (element=w886:T3)
                    n570 = call "添加设备.vi"("模式"=w884, "错误输出"=w887, "探头属性 i"=w886) -> ("error out"=w888:errorcluster, "附加信息"=w883:string, "输出有效？"=w885:bool, "探头属性 o"=w889:T3)  [unwired: 5 in]
                    n571 = Index Array(array=w901, index=w890) -> (element=w893:refnum<vi>)
                    n572 = case shown="真" w885 {
                      tunnel: w889 -> [_ w919]
                      tunnel: w902 -> [_ w910]
                      tunnel: w893 -> [_ w926]
                      tunnel: w891 -> [_ w918]
                      tunnel: w886 -> [_ w920]
                      tunnel: [w908 w923] -> w892
                      tunnel: w883 -> [w904 _]
                      frame False {
                        # "无效 或 取消不修改"
                        n573 = Empty String/Path?(string/path=w904) -> (empty?=w906:bool)
                        n574 = Select(t=" 取消", s=w906, f=w904) -> (s? t:f=w903:string)
                        n575 = Concatenate Strings("L-----------------------------------" ("字符串"), w903) -> (w908:string)
                      }
                      frame True {
                        w924 = 改动项选择."改动-探头信息"  # 改动-探头信息
                        # "有效则修改"
                        n576 = Unbundle By Name "新信息"(w919) -> ("探头地址与信息"=w921:T4)
                        n577 = Bundle By Name(cluster=w910, "改动项选择"=w924, "探测器信息"=w921) -> (w925:T41)
                        n578 = Unbundle By Name "原信息"(w920) -> ("探头地址与信息.名称"=w917:string, "探头地址与信息.网络地址"=w915:string, "探头地址与信息.备注"=w913:string)
                        n579 = Unbundle By Name "新信息"(w919) -> ("探头地址与信息.名称"=w916:string, "探头地址与信息.网络地址"=w914:string, "探头地址与信息.备注"=w912:string)
                        n580 = property class="Ctl"(reference=w926, "Value"=w925) -> ()  [unwired: 1 in, 2 out]
                        n581 = call "探头信息变更"("原地址"=w915, "原备注"=w913, "序号"=w918, "原名称"=w917, "新名称"=w916, "新地址"=w914, "新备注"=w912) -> ("Result"=w911:string)  [unwired: 7 in, 1 out]
                        n582 = Concatenate Strings("L-----------------------------------" ("字符串"), w911, "\r") -> (w923:string)
                      }
                    }
                    n583 = call "cmd启动屏幕键盘.vi"("error in (no error)"=w888, "软键盘开关"=enum16{"关闭", "打开"}."关闭") -> ()  [unwired: 8 in, 2 out]
                    n584 = Concatenate Strings("探头信息变更：\n", w892) -> (w898:string)
                    n585 = call "状态栏-插入状态信息-35点监测专用.vi"("消息内容"=w898, "状态类型"=enum16{"全部", "报警", "通信", "设置"}."设置") -> ()  [unwired: 10 in]
                  }
                  frame "修改报警设置" {
                    # "允许批量修改"
                    n586 = stacked-sequence {
                      tunnel: w932 -> [_ w936 _]
                      tunnel: w931 -> [_ w942 _]
                      tunnel: w930 -> [_ w935 _]
                      tunnel: w929 -> [_ w938 _]
                      frame #0 {
                        w933 = TRUE  # T
                        # "暂停更新列表"
                        n587 = local write "暂停更新？"(w933) -> ()
                      }
                      frame #1 {
                        w939 = 改动项选择."改动-报警限值"  # 报警限值
                        w940 = TRUE  # T
                        w949 = enum16{"单项", "批量"}."批量"  # 批量
                        w950 = enum16{"单项", "批量"}."单项"  # 单项
                        # "修改"
                        n588 = Array Size(array=w936) -> (size(s)=w952:i32)
                        n589 = Index Array(array=w936) -> (element=w947:i32)  [unwired: 1 in]
                        n590 = Index Array(array=w935, index=w947) -> (element=w945:T3)
                        n591 = Equal? "单项？"(x=w952, y=1) -> (x = y?=w946:bool)
                        n592 = Bundle By Name(cluster=w938, "改动项选择"=w939, "启用？"=w940) -> (w937:T41)
                        n593 = Select(t=w945, s=w946, f=T3 {"探头地址与信息"={"网络地址"="", "名称"="", "备注"="", "累积剂量"=0.0, "累积限值"=0.0, "硬件剂量率限值"=enum."一级限值", "剂量率限值1"=0.0, "剂量率限值2"=0.0, "报警方式"=enum."常报警"}, "测量值"={"时间"=timestamp(0 s since 1904-01-01), "数值"=0.0}, "限值"={"限值1"=0.0, "限值2"=0.0, "探头限值"=enum."一级限值"}, "探头状态"=enum."正常", "累积记录"={"起始时间"=timestamp(0 s since 1904-01-01), "结束时间"=timestamp(0 s since 1904-01-01), "累积剂量"=0.0}, "报警方式"={"报警方式"=enum."常报警", "延迟计时"=0, "报警中？"=FALSE}} ("元素")) -> (s? t:f=w943:T3)
                        n594 = Select(t=w950, s=w946, f=w949) -> (s? t:f=w948:enum16{"单项", "批量"})
                        n595 = call "修改-探头报警值-网络版.vi"("模式"=w948, "探头属性 i"=w943) -> ("取消?"=w934:bool, "探头属性 o"=w941:T3)  [unwired: 7 in, 1 out]
                        n596 = case shown="假" w934 {
                          tunnel: w942 -> [w957 _]
                          tunnel: w941 -> [w956 _]
                          tunnel: w937 -> [w955 _]
                          tunnel: w936 -> [w954 _]
                          tunnel: w935 -> [w953 _]
                          frame False {
                            # "未取消, 应用设置"
                            n597 = for {
                              tunnel: w957 -> [w964]
                              tunnel: w956 -> [w968]
                              workers-P: _ -> [_]
                              tunnel: w955 -> [w967]
                              tunnel: w954 -> [w960] mode=indexing
                              tunnel: w953 -> [w961]
                              # "必需: 网络地址"
                              # "值改变"
                              n598 = Index Array(array=w964, index=w960) -> (element=w963:refnum<vi>)
                              n599 = Index Array(array=w961, index=w960) -> (element=w959:T3)
                              n600 = Unbundle By Name(w968) -> ("探头地址与信息"=w966:T4)
                              n601 = Unbundle By Name(w959) -> ("探头地址与信息.网络地址"=w958:string)
                              n602 = Bundle By Name(cluster=w966, "网络地址"=w958) -> (w962:T4)
                              n603 = Bundle By Name(cluster=w967, "探测器信息"=w962) -> (w965:T41)
                              n604 = property class="Ctl"(reference=w963, "Value"=w965) -> ()  [unwired: 1 in, 2 out]
                            }
                          }
                          frame True {
                            # "取消修改"
                          }
                        }
                      }
                      frame #2 {
                        w969 = FALSE  # F
                        # "回复更新"
                        n605 = local write "暂停更新？"(w969) -> ()
                      }
                    }
                  }
                  frame "设备排序" {
                    # "改由单独按钮实现"
                  }
                  frame "重启累积时段" {
                    w976 = 改动项选择."动作-重启累积时段"  # 重启累积
                    # "累积剂量从现在时刻切段重启"
                    n606 = Bundle By Name(cluster=w973, "改动项选择"=w976) -> (w975:T41)
                    n607 = case shown="真" "标志-定时分段?" {
                      tunnel: w975 -> [w982 w996]
                      tunnel: w974 -> [w981 w995]
                      tunnel: w971 -> [w980 w994]
                      tunnel: w970 -> [_ w993]
                      tunnel: w971 -> [w979 _]
                      tunnel: w970 -> [_ w992]
                      frame True {
                        w977 = FALSE  # F
                        # "遍历全部"
                        n608 = Array Size(array=w979) -> (size(s)=w978:i32)
                        n609 = for {
                          N: w978 -> [_]
                          tunnel: w981 -> [w987]
                          tunnel: w982 -> [w990]
                          tunnel: w980 -> [w985]
                          workers-P: _ -> [_]
                          i -> [w983]
                          # "允许批量执行, 定时分段时所有设备都执行"
                          n610 = Index Array(array=w985, index=w983) -> (element=w984:T3)
                          n611 = Index Array(array=w987, index=w983) -> (element=w986:refnum<vi>)
                          n612 = Unbundle By Name(w984) -> ("探头地址与信息"=w989:T4)
                          n613 = Bundle By Name(cluster=w990, "探测器信息"=w989) -> (w988:T41)
                          n614 = property class="Ctl"(reference=w986, "Value"=w988) -> ()  [unwired: 1 in, 2 out]
                        }
                        n615 = local write "标志-定时分段?"(w977) -> ()
                      }
                      frame False {
                        # "遍历选中项"
                        n616 = Array Size(array=w992) -> (size(s)=w991:i32)
                        n617 = for {
                          N: w991 -> [_]
                          tunnel: w995 -> [w1001]
                          tunnel: w996 -> [w1004]
                          tunnel: w993 -> [w997] mode=indexing
                          tunnel: w994 -> [w999]
                          workers-P: _ -> [_]
                          # "允许批量执行, 定时分段时所有设备都执行"
                          n618 = Index Array(array=w999, index=w997) -> (element=w998:T3)
                          n619 = Index Array(array=w1001, index=w997) -> (element=w1000:refnum<vi>)
                          n620 = Unbundle By Name(w998) -> ("探头地址与信息"=w1003:T4)
                          n621 = Bundle By Name(cluster=w1004, "探测器信息"=w1003) -> (w1002:T41)
                          n622 = property class="Ctl"(reference=w1000, "Value"=w1002) -> ()  [unwired: 1 in, 2 out]
                        }
                      }
                    }
                  }
                  frame "累积清零" {
                    w1007 = 改动项选择."动作-累积删除"  # 累积删除
                    # "数据库操作，清空累积剂量记录和总累积剂量"
                    n623 = Bundle By Name(cluster=w1006, "改动项选择"=w1007) -> (w1005:T41)
                    n624 = for {
                      tunnel: w1010 -> [w1017] mode=indexing
                      tunnel: w1009 -> [w1026]
                      tunnel: w1008 -> [w1018]
                      tunnel: w1005 -> [w1015]
                      w1021 = DB动作类型."数据-删除数据"  # 删除数据
                      # "这里只需传入删除量"
                      # "注意: 清零操作返回值是 正无穷"
                      # "允许批量清空"
                      n625 = Index Array(array=w1026, index=w1017) -> (element=w1013:T3)
                      n626 = Index Array(array=w1018, index=w1017) -> (element=w1016:refnum<vi>)
                      n627 = Unbundle By Name(w1013) -> ("探头地址与信息.名称"=w1025:string)
                      n628 = Bundle By Name(cluster=T27 {"名称"="", "多条记录(空则全删)"=[]}, "名称"=w1025) -> (w1020:T27)
                      n629 = Bundle By Name(cluster=T28 {"动作类型"=enum."DB-加载设备", "输入数据"=variant} ("DB动作集"), "动作类型"=w1021, "输入数据"=w1020) -> (w1022:T28)
                      n630 = call "TOP-累积剂量数据管理.vi"("DB动作集"=w1022) -> ("输出数据"=w1019:variant)  [unwired: 9 in, 1 out]
                      n631 = Variant To Data(type=0.0, Variant=w1019) -> (data=w1011:dbl)  [unwired: 1 in, 1 out]
                      n632 = Bundle By Name(cluster=w1015, "探测器信息.累积剂量"=w1011) -> (w1014:T41)
                      n633 = property class="Ctl"(reference=w1016, "Value"=w1014) -> ()  [unwired: 1 in, 2 out]
                    }
                  }
                  frame "添加设备" {
                    # "添加设备，输入空属性，输出新的无冲突属性，然后创建添加通信单元"
                    n634 = stacked-sequence {
                      frame #0 {
                        # "创建与扫描询问窗口"
                      }
                      frame #1 {
                        n635 = call "弹窗-创建设备选项.vi"() -> ("初始化的属性"=w1027:T3[])  [unwired: 11 in]
                        n636 = for {
                          tunnel: w1027 -> [w1028] mode=indexing
                          # "批量创建"
                          n637 = stacked-sequence {
                            seq-local: [w1032 _] -> [_ w1041]
                            seq-local: [w1031 _] -> [_ w1042]
                            tunnel: w1028 -> [w1029 _]
                            frame #0 {
                              w1030 = enum16{"新建设备", "编辑设备"}."新建设备"  # 新建
                              # "数据库中添加设备"
                              n638 = call "添加设备.vi"("模式"=w1030, "探头属性 i"=w1029) -> ("输出有效？"=w1033:bool, "探头属性 o"=w1032:T3)  [unwired: 6 in, 2 out]
                              n639 = case shown="真" w1033 {
                                tunnel: w1032 -> [_ w1037]
                                tunnel: [w1034 w1035] -> w1031
                                frame False {
                                w1034 = errorcluster {"status"=TRUE, "code"=0, "source"=""}  # 错误
                                # "无效"
                                }
                                frame True {
                                w1040 = DB动作类型."设备-登记新设备+数据表"  # 新设备
                                # "有效，则在数据库中添加"
                                n640 = Unbundle By Name(w1037) -> ("探头地址与信息"=w1036:T4)
                                n641 = Bundle By Name(cluster=T28 {"动作类型"=enum."设备-删除设备", "输入数据"=variant(string "192.168.1.200:200")} ("DB动作集"), "动作类型"=w1040, "输入数据"=w1036) -> (w1039:T28)
                                n642 = call "TOP-累积剂量数据管理.vi"("DB动作集"=w1039) -> ("error out"=w1035:errorcluster)  [unwired: 9 in, 1 out]
                                }
                              }
                            }
                            frame #1 {
                              # "添加通信单元"
                              n643 = case shown="无错误" w1042 {
                                tunnel: w1041 -> [w1043 _]
                                frame No Error {
                                # "有效且数据库添加成功 , 确认添加设备"
                                n644 = stacked-sequence {
                                seq-local: [w1048 _ _] -> [_ w1060 _]
                                seq-local: [w1045 _ _] -> [_ _ _]
                                seq-local: [w1047 _ _] -> [_ w1059 _]
                                seq-local: [w1046 _ _] -> [_ w1058 _]
                                seq-local: [_ w1056 _] -> [_ _ w1067]
                                tunnel: w1043 -> [w1049 _ w1075]
                                frame #0 {
                                w1055 = 128  # 重入运行
                                # "创建“通信单元”实例"
                                n645 = vi-ref "探头通信模块.vi"() -> (w1050:refnum<vi>)
                                n646 = property class="VI接口类型5"(reference=w1050) -> (reference out=w1044:refnum<vi>, "Name"=w1054:string)  [unwired: 1 in, 1 out]
                                n647 = Open VI Reference(type specifier VI Refnum (for type only)=w1044, vi path=w1054, options=w1055) -> (vi reference=w1051:refnum<vi>)  [unwired: 3 in, 1 out]
                                n648 = call-by-ref "开始异步调用"(reference=w1051, "探头属性"=w1049) -> (reference out=w1048:refnum<vi>)  [unwired: 12 in, 1 out]
                                n649 = call "通过控件名获取控件引用.vi"("控件名数组"=string[] ["停止", "改动项", "探头属性"], "VI引用"=w1048) -> ("控件引用输出"=w1052:refnum<vi>[])  [unwired: 7 in, 2 out]
                                n650 = Index Array(array=w1052) -> (element #1=w1045:refnum<vi>, element #2=w1047:refnum<vi>, element #3=w1046:refnum<vi>)  [unwired: 3 in]
                                }
                                frame #1 {
                                # "添加引用"
                                n651 = local read "通信单元-探头属性引用[]"() -> (w1064:refnum<vi>[])
                                n652 = local read "通信单元-改动项引用[]"() -> (w1063:refnum<vi>[])
                                n653 = local read "通信单元-VI引用[]"() -> (w1065:refnum<vi>[])
                                n654 = Insert Into Array(array=w1065, new element=w1060) -> (w1061:refnum<vi>[])  [unwired: 1 in]
                                n655 = Insert Into Array(array=w1063, new element=w1059) -> (w1062:refnum<vi>[])  [unwired: 1 in]
                                n656 = Insert Into Array(array=w1064, new element=w1058) -> (w1057:refnum<vi>[])  [unwired: 1 in]
                                n657 = Array Size(array=w1057) -> (size(s)=w1056:i32)
                                n658 = local write "通信单元-改动项引用[]"(w1062) -> ()
                                n659 = local write "通信单元-探头属性引用[]"(w1057) -> ()
                                n660 = local write "通信单元-VI引用[]"(w1061) -> ()
                                }
                                frame #2 {
                                w1072 = enum16{"全部", "报警", "通信", "设置"}."设置"  # 设置
                                # "状态栏提示"
                                n661 = Unbundle By Name(w1075) -> ("探头地址与信息.名称"=w1074:string, "探头地址与信息.网络地址"=w1073:string)
                                n662 = local read "监测数量限值"() -> (w1070:cluster{"min":i32, "max":i32})
                                n663 = call "创建文本"("探头名称"=w1074, "地址"=w1073) -> ("Result"=w1071:string)  [unwired: 12 in, 1 out]
                                n664 = Unbundle By Name(w1070) -> ("max"=w1069:i32, "min"=w1068:i32)
                                n665 = In Range and Coerce(upper limit=w1069, x=w1067, lower limit=w1068) -> (In Range?=w1066:bool)  [unwired: 1 out]
                                n666 = case shown="假" w1066 {
                                selector: w1066 -> [w1077 _]
                                frame False {
                                # "超出范围，停止监测VI"
                                n667 = local read "监-停止信号"() -> (w1078:refnum<vi>)
                                n668 = property class="Ctl"(reference=w1078, "Val(Sgnl)"=w1077) -> (error out=w1076:errorcluster)  [unwired: 1 in, 1 out]
                                n669 = call <vilib>:"Clear Errors.vi"("error in (no error)"=w1076) -> ()  [unwired: 5 in, 2 out]
                                }
                                frame True {
                                # "范围内，不停止监测VI"
                                }
                                }
                                n670 = call "状态栏-插入状态信息-35点监测专用.vi"("消息内容"=w1071, "状态类型"=w1072) -> ()  [unwired: 10 in]
                                }
                                }
                                }
                                frame Error {
                                # "无效 或 取消添加设备"
                                }
                              }
                            }
                          }
                        }
                      }
                    }
                  }
                  frame "删除设备" {
                    n671 = stacked-sequence {
                      seq-local: [w1085 _ _] -> [_ w1112 _]
                      seq-local: [w1084 _ _] -> [_ _ w1150]
                      seq-local: [_ w1110 _] -> [_ _ w1139]
                      tunnel: w1080 -> [w1088 w1111 _]
                      tunnel: w1079 -> [w1087 _ _]
                      frame #0 {
                        # "确认对话框"
                        n672 = for "For循环" {
                          N -> [w1109]
                          tunnel: w1088 -> [w1100] mode=indexing
                          tunnel: w1087 -> [w1107]
                          shift-right: [w1095] -> w1084
                          shift-left: "" -> [w1097]
                          tunnel: T28 {"动作类型"=enum."DB-文件初始化+连接", "输入数据"=variant} ("DB动作集") -> [w1093]
                          i -> [w1108]
                          # "构建-删除清单"
                          n673 = Decrement(x=w1109) -> (x-1=w1105:i32)
                          n674 = Equal?(x=w1105, y=w1108) -> (x = y?=w1104:bool)
                          n675 = Index Array(array=w1107, index=w1100) -> (element=w1106:T3)
                          n676 = Increment(x=w1100) -> (x+1=w1094:i32)
                          n677 = Unbundle By Name(w1106) -> ("探头地址与信息.网络地址"=w1091:string, "探头地址与信息.名称"=w1099:string)
                          n678 = Select(t="", s=w1104, f="\r\n") -> (s? t:f=w1101:string)
                          n679 = Bundle By Name(cluster=w1093, "动作类型"=DB动作类型."设备-删除设备", "输入数据"=w1091) -> (w1090:T28)
                          n680 = call "构建探头信息"("探头号"=w1094, "探头信息"=w1099) -> ("Result"=w1098:string)  [unwired: 12 in, 1 out]
                          n681 = Concatenate Strings(w1098, w1101) -> (w1096:string)
                          n682 = call "TOP-累积剂量数据管理.vi"("DB动作集"=w1090) -> ("error out"=w1089:errorcluster)  [unwired: 9 in, 1 out]
                          n683 = call <vilib>:"Simple Error Handler.vi"("error in (no error)"=w1089) -> ()  [unwired: 4 in, 5 out]
                          n684 = Concatenate Strings(w1097, w1096) -> (w1095:string)
                        }
                        n685 = Concatenate Strings("删除设备？\n" ("字符串"), w1084) -> (w1082:string)
                        n686 = call "将删除以下设备"("Message"=w1082) -> ("删除"=w1085:bool)  [unwired: 9 in, 1 out]
                      }
                      frame #1 {
                        # "删除设备"
                        n687 = case shown="真" w1112 {
                          tunnel: w1111 -> [w1114 w1123]
                          tunnel: [w1113 w1115] -> w1110
                          frame False {
                            # "取消"
                            n688 = Array Size(array=w1114) -> (size(s)=w1113:i32)
                          }
                          frame True {
                            # "删除"
                            n689 = local read "通信单元-探头属性引用[]"() -> (w1120:refnum<vi>[])
                            n690 = local read "通信单元-改动项引用[]"() -> (w1121:refnum<vi>[])
                            n691 = local read "通信单元-VI引用[]"() -> (w1122:refnum<vi>[])
                            n692 = Reverse 1D Array(array=w1123) -> (reversed array=w1119:i32[])
                            n693 = for "For循环" {
                              tunnel: w1119 -> [w1136] mode=indexing
                              shift-right: [w1131] -> w1116
                              shift-left: w1122 -> [w1135]
                              shift-right: [w1130] -> w1118
                              shift-left: w1121 -> [w1134]
                              shift-right: [w1129] -> w1117
                              shift-left: w1120 -> [w1133]
                              # "删除引用，关闭实例"
                              n694 = Delete From Array(array=w1135, index=w1136) -> (deleted portion=w1132:refnum<vi>, array with subset deleted=w1131:refnum<vi>[])  [unwired: 1 in]
                              n695 = invoke class="VI (严格)" method="Abort VI"(reference=w1132) -> (reference out=w1127:refnum<vi>, error out=w1125:errorcluster)  [unwired: 2 in, 1 out]
                              n696 = Delete From Array(array=w1134, index=w1136) -> (array with subset deleted=w1130:refnum<vi>[])  [unwired: 1 in, 1 out]
                              n697 = Delete From Array(array=w1133, index=w1136) -> (array with subset deleted=w1129:refnum<vi>[])  [unwired: 1 in, 1 out]
                              n698 = invoke class="VI (严格)" method="FP.Close"(reference=w1127, error in=w1125) -> (reference out=w1126:refnum<vi>, error out=w1124:errorcluster)  [unwired: 1 in, 1 out]
                              n699 = Close Reference(reference=w1126, error in (no error)=w1124) -> (error out=w1128:errorcluster)
                              n700 = call <vilib>:"Clear Errors.vi"("error in (no error)"=w1128) -> ()  [unwired: 5 in, 2 out]
                            }
                            n701 = local write "通信单元-VI引用[]"(w1116) -> ()
                            n702 = local write "通信单元-改动项引用[]"(w1118) -> ()
                            n703 = local write "通信单元-探头属性引用[]"(w1117) -> ()
                            n704 = Array Size(array=w1116) -> (size(s)=w1115:i32)
                          }
                        }
                      }
                      frame #2 {
                        w1145 = enum16{"全部", "报警", "通信", "设置"}."设置"  # 设置
                        w1151 = TRUE  # T
                        # "状态栏提示，列表回到顶部（删除超过一页时需要）"
                        n705 = local read "监测数量限值"() -> (w1142:cluster{"min":i32, "max":i32})
                        n706 = Unbundle By Name(w1142) -> ("max"=w1141:i32, "min"=w1140:i32)
                        n707 = Search and Replace String(replace all?=w1151, input string=w1150, search string="\r\n", replace string="，") -> (result string=w1147:string)  [unwired: 4 in, 3 out]
                        n708 = Concatenate Strings("已移除设备：", w1147) -> (w1144:string)
                        n709 = In Range and Coerce(upper limit=w1141, x=w1139, lower limit=w1140) -> (In Range?=w1138:bool)  [unwired: 1 out]
                        n710 = case shown="假" w1138 {
                          selector: w1138 -> [w1153 _]
                          frame False {
                            # "超出范围，停止监测VI"
                            n711 = local read "监-停止信号"() -> (w1154:refnum<vi>)
                            n712 = property class="Ctl"(reference=w1154, "Val(Sgnl)"=w1153) -> (error out=w1152:errorcluster)  [unwired: 1 in, 1 out]
                            n713 = call <vilib>:"Clear Errors.vi"("error in (no error)"=w1152) -> ()  [unwired: 5 in, 2 out]
                          }
                          frame True {
                            # "范围内，不停止监测VI"
                          }
                        }
                        n714 = call "状态栏-插入状态信息-35点监测专用.vi"("消息内容"=w1144, "状态类型"=w1145) -> ()  [unwired: 10 in]
                        n715 = property on="实时数据列表" class="MCListbox (严格)"("TopLeft"=T15 {"Row"=0, "Column"=0} ("左上可见单元格"), "Val(Sgnl)"=i32[] [] ("实时数据列表")) -> ()  [unwired: 2 in, 2 out]
                      }
                    }
                  }
                  frame "累积定时" {
                    # "设置累积分段定时"
                    n716 = vi-ref "弹窗-设置周期.vi"() -> (w1157:refnum<vi>)
                    n717 = property class="VI接口类型0"(reference=w1157) -> (reference out=w1155:refnum<vi>, "Name"=w1159:string)  [unwired: 1 in, 1 out]
                    n718 = Open VI Reference(type specifier VI Refnum (for type only)=w1155, vi path=w1159, options=128 ("选项")) -> (vi reference=w1156:refnum<vi>)  [unwired: 3 in, 1 out]
                    n719 = call-by-ref "开始异步调用"(reference=w1156) -> ()  [unwired: 13 in, 2 out]
                  }
                }
              }
              frame True {
                # "不产生菜单事件"
              }
            }
            n720 = flat-sequence {
              tunnel: w814 -> [_]
              frame #0 {
                w820 = FALSE  # F
                n721 = local write "菜单锁-设备表"(w820) -> ()
              }
            }
          }
          event Value Change {
            # "报警列表，菜单事件处理"
            n722 = event-data() -> ("CtlRef"=w1164:refnum<vi>)  [unwired: 1 in, 5 out]
            n723 = flat-sequence {
              tunnel: [w1166] -> w1161
              frame #0 {
                w1166 = TRUE  # T
                n724 = local write "菜单锁-报警表"(w1166) -> ()
              }
            }
            n725 = local read "点到行列-报警记录"() -> (w1163:T14)
            n726 = local read "暂停更新？"() -> (w1162:bool)
            n727 = case shown="假" w1162 {
              tunnel: w1164 -> [w1173 _]
              tunnel: w1163 -> [w1171 _]
              tunnel: w1161 -> [w1167 _]
              tunnel: [w1167 _] -> w1160
              frame False {
                # "非暂停，可执行"
                n728 = local read "报警记录缓存数据文件"() -> (w1170:string[])
                n729 = local read "报警记录列表"() -> (w1168:i32[])
                n730 = property class="Enum (严格)"(reference=w1173) -> ("RingText.Text"=w1172:string)  [unwired: 1 in, 2 out]
                n731 = Unbundle By Name(w1171) -> ()  [unwired: 1 out]
                n732 = for "For循环" {
                  tunnel: w1170 -> [w1176]
                  tunnel: [w1175] -> w1169 mode=indexing
                  tunnel: w1168 -> [w1174] mode=indexing
                  workers-P: _ -> [_]
                  n733 = Index Array(array=w1176, index=w1174) -> (element=w1175:string)
                }
                n734 = case shown="\"预览并生成报表\"" w1172 {
                  tunnel: w1169 -> [_ _ w1208 w1244 _]
                  tunnel: w1168 -> [_ _ w1205 _ w1278]
                  frame "假", Default {
                  }
                  frame "刷新" {
                    # "刷新报警记录清单"
                    n735 = call "读取-缓存数据文件夹至报警记录列表-网络版.vi"() -> ("文件名"=→"报警记录缓存数据文件":string[], "新记录文件名"=w1189:string[], "新记录列表"=w1190:string[][], "报警记录列表"=w1185:string[][])  [unwired: 8 in]
                    n736 = Array Size(array=w1185) -> (size(s)=w1193:i32[])
                    n737 = for {
                      workers-P: _ -> [_]
                      tunnel: w1190 -> [w1200] mode=indexing
                      tunnel: w1189 -> [w1199] mode=indexing
                      tunnel: [w1198] -> w1191 mode=indexing
                      # "数组到簇绑定"
                      n738 = Bundle("新记录列表"=w1200, "字符串"=w1199) -> (w1198:cluster{"新记录列表":string[], "字符串":string})  [unwired: 1 in]
                    }
                    n739 = Index Array(array=w1193) -> (element=w1192:i32)  [unwired: 1 in]
                    n740 = local write "报警记录数"(w1192) -> ()
                    n741 = for {
                      tunnel: [w1197] -> w1180 mode=indexing
                      workers-P: _ -> [_]
                      tunnel: w1185 -> [_] mode=indexing
                      i -> [w1197]
                    }
                    n742 = property on="新记录簇" class="Arr (严格)"("Val(Sgnl)"=w1191) -> ()  [unwired: 2 in, 2 out]
                    n743 = Increment(x=w1180) -> (x+1=w1184:i32[])
                    n744 = Number To Decimal String(number=w1184) -> (decimal integer string=w1187:string[])  [unwired: 1 in]
                    n745 = Array Size(array=w1180) -> (size(s)=w1183:i32)
                    n746 = property on="报警记录列表" class="MCListbox (严格)"() -> (error out=w1177:errorcluster, "ColHdrString"=w1179:string[])  [unwired: 2 in, 1 out]
                    n747 = Number To Decimal String(number=w1183) -> (decimal integer string=w1182:string)  [unwired: 1 in]
                    n748 = Insert Into Array(array=w1185, index (col)=0 ("禁用的索引 (列)"), new element=w1187) -> (w1186:string[][])  [unwired: 1 in]
                    n749 = Replace Array Subset(array=w1179, new element=w1182, index=0 ("索引")) -> (w1178:string[])
                    n750 = property on="报警记录列表" class="MCListbox (严格)"(error in=w1177, "ColHdrString"=w1178, "ItemNames"=w1186, "Val(Sgnl)"=i32[] [] ("报警记录列表"), "TopLeft"=T15 {"Row"=0, "Column"=0} ("左上可见单元格")) -> ()  [unwired: 1 in, 2 out]
                  }
                  frame "预览并生成报表" {
                    # "避免空选"
                    # "获得文件路径，预览并生成报表"
                    n751 = property on="报警记录列表" class="MCListbox (严格)"() -> ("ItemNames"=w1206:string[][])  [unwired: 2 in, 2 out]
                    n752 = Index Array(array=w1205) -> (element=w1204:i32)  [unwired: 1 in]
                    n753 = Increment(x=w1204) -> (x+1=w1202:i32)
                    n754 = Array Size(array=w1206) -> (size(s)=w1207:i32[])
                    n755 = Index Array(array=w1207) -> (element=w1203:i32)  [unwired: 1 in]
                    n756 = Greater Or Equal? "有效行？"(x=w1203, y=w1202) -> (x >= y?=w1201:bool)
                    n757 = case shown="真" w1201 {
                      tunnel: w1208 -> [_ w1209]
                      frame False {
                      }
                      frame True {
                        # "有效行"
                        n758 = call "路径查找创建-报警记录清单-网络版.vi"() -> ("缓存数据文件夹"=w1210:path)  [unwired: 2 in, 13 out]
                        n759 = vi-ref "通用报警记录浏览.vi"() -> (w1211:refnum<vi>)
                        n760 = disable-structure shown="禁用" {
                          disable-tunnel: w1211 -> [w1214 w1240]
                          disable-tunnel: w1210 -> [w1213 w1241]
                          disable-tunnel: w1209 -> [w1212 w1243]
                          frame Disabled {
                            # "预分配重入"
                            n761 = for "For循环" {
                              tunnel: w1214 -> [w1221]
                              tunnel: w1213 -> [w1217]
                              tunnel: w1212 -> [w1215] mode=indexing
                              # "打开多个窗口？"
                              n762 = property class="VI"(reference=w1221) -> ("Name"=w1220:string)  [unwired: 1 in, 2 out]
                              n763 = Build Path(base path=w1217, name or relative path=w1215) -> (appended path=w1216:path)
                              n764 = Open VI Reference(type specifier VI Refnum (for type only)=refnum<vi> refnum ("类型说明符VI引用句柄（仅用于类型）"), vi path=w1220, options=128 ("选项")) -> (vi reference=w1218:refnum<vi>)  [unwired: 3 in, 1 out]
                              n765 = call-by-ref "开始异步调用"(reference=w1218, "缓存数据路径"=w1216) -> ()  [unwired: 12 in, 2 out]
                            }
                          }
                          frame Enabled {
                            # "共享副本重入"
                            n766 = Index Array(array=w1243) -> (element=w1242:string)  [unwired: 1 in]
                            n767 = Build Path(base path=w1241, name or relative path=w1242) -> (appended path=w1233:path)
                            n768 = invoke class="VI" method="FP.Open"(reference=w1240, "Activate"=TRUE ("激活？"), "State"=T18."Hidden" ("状态")) -> (reference out=w1237:refnum<vi>, error out=w1224:errorcluster)  [unwired: 2 in, 3 out]
                            n769 = call "通过控件名获取控件引用.vi"("控件名数组"=string[] ["缓存数据路径"], "VI引用"=w1237) -> ("控件引用输出"=w1235:refnum<vi>[], "VI引用o"=w1232:refnum<vi>)  [unwired: 7 in, 1 out]
                            n770 = Index Array(array=w1235) -> (element=w1234:refnum<vi>)  [unwired: 1 in]
                            n771 = property class="Ctl"(reference=w1234, error in=w1224, "Val(Sgnl)"=w1233) -> (error out=w1223:errorcluster)  [unwired: 1 out]
                            n772 = invoke class="VI" method="Run VI"(reference=w1232, error in=w1223, "Wait until done"=FALSE ("结束前等待"), "Auto Dispose Ref"=TRUE ("自动销毁引用")) -> (reference out=w1229:refnum<vi>, error out=w1228:errorcluster)  [unwired: 1 in, 3 out]
                            n773 = invoke class="VI" method="FP.Open"(reference=w1229, error in=w1228, "Activate"=TRUE ("激活？"), "State"=T18."Standard" ("状态")) -> (error out=w1225:errorcluster)  [unwired: 1 in, 4 out]
                            n774 = call <vilib>:"Clear Errors.vi"("error in (no error)"=w1225) -> ()  [unwired: 5 in, 2 out]
                          }
                        }
                      }
                    }
                  }
                  frame "删除记录" {
                    # "删除缓存的xml文件，然后刷新"
                    n775 = stacked-sequence {
                      seq-local: [w1245 _ _ _] -> [_ _ w1252 _]
                      seq-local: [_ w1251 _ _] -> [_ _ w1253 _]
                      tunnel: w1244 -> [w1246 _ _ _]
                      frame #0 {
                        # "删除缓存数据xml文件"
                        n776 = call "路径查找创建-报警记录清单-网络版.vi"() -> ("缓存数据文件夹"=w1247:path)  [unwired: 2 in, 13 out]
                        n777 = for "For循环" {
                          tunnel: w1247 -> [w1250]
                          tunnel: w1246 -> [w1249] mode=indexing
                          tunnel: [w1248] -> w1245 mode=indexing
                          workers-P: _ -> [_]
                          n778 = Build Path(base path=w1250, name or relative path=w1249) -> (appended path=w1248:path)
                        }
                      }
                      frame #1 {
                        # "弹窗确认"
                        n779 = call "显示对话框信息"() -> ("确定"=w1251:bool)  [unwired: 10 in, 1 out]
                      }
                      frame #2 {
                        # "删除操作"
                        n780 = case shown="真" w1253 {
                          tunnel: w1252 -> [_ w1254]
                          frame False {
                          }
                          frame True {
                            n781 = for "For循环" {
                              tunnel: w1254 -> [w1256] mode=indexing
                              n782 = Delete(path (use dialog)=w1256) -> (error out=w1255:errorcluster)  [unwired: 4 in, 2 out]
                              n783 = call <vilib>:"Clear Errors.vi"("error in (no error)"=w1255) -> ()  [unwired: 5 in, 2 out]
                            }
                          }
                        }
                      }
                      frame #3 {
                        # "刷新列表"
                        n784 = call "读取-缓存数据文件夹至报警记录列表-网络版.vi"() -> ("文件名"=w1270:string[], "报警记录列表"=w1265:string[][])  [unwired: 8 in, 2 out]
                        n785 = property on="报警记录列表" class="MCListbox (严格)"() -> ("ColHdrString"=w1259:string[])  [unwired: 2 in, 2 out]
                        n786 = for {
                          tunnel: [w1271] -> w1260 mode=indexing
                          workers-P: _ -> [_]
                          tunnel: w1265 -> [_] mode=indexing
                          i -> [w1271]
                        }
                        n787 = local write "报警记录缓存数据文件"(w1270) -> ()
                        n788 = Increment(x=w1260) -> (x+1=w1264:i32[])
                        n789 = Array Size(array=w1260) -> (size(s)=w1263:i32)
                        n790 = Number To Decimal String(number=w1264) -> (decimal integer string=w1267:string[])  [unwired: 1 in]
                        n791 = Number To Decimal String(number=w1263) -> (decimal integer string=w1262:string)  [unwired: 1 in]
                        n792 = Insert Into Array(array=w1265, index (col)=0 ("禁用的索引 (列)"), new element=w1267) -> (w1266:string[][])  [unwired: 1 in]
                        n793 = Replace Array Subset(array=w1259, new element=w1262, index=0 ("索引")) -> (w1258:string[])
                        n794 = property on="报警记录列表" class="MCListbox (严格)"("ColHdrString"=w1258, "ItemNames"=w1266, "Val(Sgnl)"=i32[] [] ("报警记录列表"), "TopLeft"=T15 {"Row"=0, "Column"=0} ("左上可见单元格")) -> ()  [unwired: 2 in, 2 out]
                      }
                    }
                  }
                  frame "复制选中项至剪贴板" {
                    w1274 = 0 ("禁用的索引 (列)")
                    # "复制选中行到剪贴板"
                    n795 = property on="报警记录列表" class="多列列表框 (严格)"() -> ("ItemNames"=w1276:string[][], "ColHdrString"=w1273:string[])  [unwired: 2 in, 2 out]
                    n796 = Delete From Array(array=w1276, index (col)=w1274) -> (array with subset deleted=w1275:string[][])  [unwired: 2 in, 1 out]
                    n797 = Delete From Array(array=w1273, index=w1274) -> (array with subset deleted=w1272:string[])  [unwired: 1 in, 1 out]
                    n798 = for {
                      tunnel: w1275 -> [w1293] mode=indexing
                      tunnel: [w1294] -> w1282 mode=indexing
                      tunnel: [w1293] -> w1284
                      n799 = To Variant(anything=w1293) -> (Variant=w1294:variant)
                    }
                    n800 = call "状态栏-插入状态信息-35点监测专用.vi"("消息内容"="已复制 报警记录列表选中项 至剪贴板", "状态类型"=enum16{"全部", "报警", "通信", "设置"}."设置") -> ()  [unwired: 10 in]
                    n801 = call "重排数组.vi"("新索引顺序"=w1278, "原数组"=w1282) -> ("排序后数组"=w1283:variant[])  [unwired: 9 in]
                    n802 = for {
                      tunnel: w1283 -> [w1292] mode=indexing
                      tunnel: w1284 -> [w1291]
                      tunnel: [w1290] -> w1285 mode=indexing
                      n803 = Variant To Data(type=w1291, Variant=w1292) -> (data=w1290:string[])  [unwired: 1 in, 1 out]
                    }
                    n804 = Array To Spreadsheet String(array=w1285, 3:"%s" ("格式字符串")) -> (spreadsheet string=w1288:string)  [unwired: 1 in]
                    n805 = Array To Spreadsheet String(array=w1272, 3:"%s" ("格式字符串")) -> (spreadsheet string=w1277:string)  [unwired: 1 in]
                    n806 = control-ref of="本应用程序"() -> (w1287:refnum<vi>)
                    n807 = Concatenate Strings(w1277, w1288) -> (w1289:string)
                    n808 = invoke class="App" method="Clipboard.Write"(reference=w1287, "Param 0"=w1289) -> ()  [unwired: 2 in, 4 out]
                  }
                }
              }
              frame True {
                # "暂停发送，不执行"
              }
            }
            n809 = flat-sequence {
              tunnel: w1160 -> [_]
              frame #0 {
                w1165 = FALSE  # F
                n810 = local write "菜单锁-报警表"(w1165) -> ()
              }
            }
          }
          event "设备排序": Value Change {
            n811 = event-data() -> ("NewVal"=w1295:bool)  [unwired: 1 in, 5 out]
            n812 = case shown="真" w1295 {
              frame False {
                # "点击  结束修改"
                n813 = property on="实时数据列表" class="MCListbox (严格)"() -> ("ItemNames"=w1298:string[][])  [unwired: 2 in, 2 out]
                n814 = Index Array "探头序号咧"(array=w1298, index (col)=0 ("禁用的索引 (列)")) -> (element=w1299:string[])  [unwired: 1 in]
                n815 = Decimal String To Number(string=w1299) -> (number=w1300:i32[])  [unwired: 2 in, 1 out]
                n816 = Decrement(x=w1300) -> (x-1=w1296:i32[])
                n817 = stacked-sequence {
                  seq-local: [w1301 _ _] -> [_ w1306 w1351]
                  tunnel: w1296 -> [w1302 w1307 _]
                  frame #0 {
                    w1303 = DB动作类型."设备-重排"  # 重排设备
                    # "数据库动作, 重排设备列表"
                    n818 = Bundle By Name(cluster=T28 {"动作类型"=enum."DB-文件初始化+连接", "输入数据"=variant} ("DB动作集"), "动作类型"=w1303, "输入数据"=w1302) -> (w1304:T28)
                    n819 = call "TOP-累积剂量数据管理.vi"("DB动作集"=w1304) -> ("error out"=w1301:errorcluster)  [unwired: 9 in, 1 out]
                  }
                  frame #1 {
                    # "更改受影响的项"
                    n820 = case shown="无错误" w1306 {
                      tunnel: w1307 -> [w1308 _]
                      frame No Error {
                        # "注意：不要出现空的行"
                        n821 = local read "通信单元-探头属性引用[]"() -> (w1313:refnum<vi>[])
                        n822 = local read "通信单元-改动项引用[]"() -> (w1312:refnum<vi>[])
                        n823 = local read "通信单元-VI引用[]"() -> (w1314:refnum<vi>[])
                        n824 = stacked-sequence "依次重排" {
                          tunnel: w1314 -> [w1320 _ _]
                          tunnel: w1313 -> [_ w1327 _]
                          tunnel: w1312 -> [_ _ w1339]
                          tunnel: w1308 -> [w1318 w1330 w1341]
                          tunnel: [w1316 _ _] -> w1311
                          tunnel: [_ w1328 _] -> w1310
                          tunnel: [_ _ w1338] -> w1309
                          frame #0 {
                            n825 = for "For循环" {
                              workers-P: _ -> [_]
                              tunnel: w1320 -> [w1324] mode=indexing
                              tunnel: [w1325] -> w1319 mode=indexing
                              tunnel: [w1324] -> w1315
                              n826 = To Variant(anything=w1324) -> (Variant=w1325:variant)
                            }
                            n827 = call "重排数组.vi"("新索引顺序"=w1318, "原数组"=w1319) -> ("排序后数组"=w1317:variant[])  [unwired: 9 in]
                            n828 = for "For循环" {
                              workers-P: _ -> [_]
                              tunnel: w1317 -> [w1323] mode=indexing
                              tunnel: [w1322] -> w1316 mode=indexing
                              tunnel: w1315 -> [w1321]
                              n829 = Variant To Data(type=w1321, Variant=w1323) -> (data=w1322:refnum<vi>)  [unwired: 1 in, 1 out]
                            }
                          }
                          frame #1 {
                            n830 = for "For循环" {
                              workers-P: _ -> [_]
                              tunnel: w1327 -> [w1335] mode=indexing
                              tunnel: [w1336] -> w1331 mode=indexing
                              tunnel: [w1335] -> w1326
                              n831 = To Variant(anything=w1335) -> (Variant=w1336:variant)
                            }
                            n832 = call "重排数组.vi"("新索引顺序"=w1330, "原数组"=w1331) -> ("排序后数组"=w1329:variant[])  [unwired: 9 in]
                            n833 = for "For循环" {
                              workers-P: _ -> [_]
                              tunnel: w1329 -> [w1334] mode=indexing
                              tunnel: [w1333] -> w1328 mode=indexing
                              tunnel: w1326 -> [w1332]
                              n834 = Variant To Data(type=w1332, Variant=w1334) -> (data=w1333:refnum<vi>)  [unwired: 1 in, 1 out]
                            }
                          }
                          frame #2 {
                            n835 = for "For循环" {
                              workers-P: _ -> [_]
                              tunnel: w1339 -> [w1346] mode=indexing
                              tunnel: [w1347] -> w1342 mode=indexing
                              tunnel: [w1346] -> w1337
                              n836 = To Variant(anything=w1346) -> (Variant=w1347:variant)
                            }
                            n837 = call "重排数组.vi"("新索引顺序"=w1341, "原数组"=w1342) -> ("排序后数组"=w1340:variant[])  [unwired: 9 in]
                            n838 = for "For循环" {
                              workers-P: _ -> [_]
                              tunnel: w1340 -> [w1345] mode=indexing
                              tunnel: [w1344] -> w1338 mode=indexing
                              tunnel: w1337 -> [w1343]
                              n839 = Variant To Data(type=w1343, Variant=w1345) -> (data=w1344:refnum<vi>)  [unwired: 1 in, 1 out]
                            }
                          }
                        }
                        n840 = local write "通信单元-VI引用[]"(w1311) -> ()
                        n841 = local write "通信单元-探头属性引用[]"(w1310) -> ()
                        n842 = local write "通信单元-改动项引用[]"(w1309) -> ()
                      }
                      frame Error {
                      }
                    }
                  }
                  frame #2 {
                    w1352 = FALSE  # F
                    w1354 = FALSE  # F
                    # "更改标志，使在状态机中检测到更改，状态栏提示"
                    n843 = local write "暂停更新？"(w1354) -> ()
                    n844 = property on="实时数据列表" class="多列列表框 (严格)"("Allow Drop"=w1352, "Allow Item Drag"=w1352) -> ()  [unwired: 2 in, 2 out]
                    n845 = Select(t="数据库排序出错, 重启软件查看效果, 必要时重新添加设备" ("消息内容"), s=w1351, f="探头排序完成" ("消息内容")) -> (s? t:f=w1348:string)
                    n846 = call "状态栏-插入状态信息-35点监测专用.vi"("消息内容"=w1348, "状态类型"=enum16{"全部", "报警", "通信", "设置"}."设置") -> ()  [unwired: 10 in]
                  }
                }
              }
              frame True {
                # "开始排序"
                n847 = flat-sequence {
                  frame #0 {
                    w1355 = TRUE  # T
                    # "暂停更新，启动动态效果"
                    n848 = local write "暂停更新？"(w1355) -> ()
                  }
                  frame #1 {
                    w1356 = TRUE  # T
                    # "进入编辑模式"
                    n849 = property on="实时数据列表" class="多列列表框 (严格)"("Allow Drop"=w1356, "Allow Item Drag"=w1356) -> ()  [unwired: 2 in, 2 out]
                  }
                  frame #2 {
                    # "状态栏提示"
                    n850 = call "状态栏-插入状态信息-35点监测专用.vi"("消息内容"="**操作提示：对当前闪烁的列表“行”拖拽排序，按菜单栏左侧按钮可结束排序。", "状态类型"=enum16{"全部", "报警", "通信", "设置"}."设置") -> ()  [unwired: 10 in]
                  }
                }
              }
            }
          }
          event "新记录？": Value Change {
            # "刷新列表"
            n851 = event-data() -> ()  [unwired: 1 in, 6 out]
            n852 = property on="菜单项-报警列表" class="Enum (严格)"("Val(Sgnl)"=enum16{"刷新", "预览并生成报表", "删除记录"}."刷新" ("菜单项-报警列表")) -> ()  [unwired: 2 in, 2 out]
          }
          event "设置": Value Change {
            (unwired) FALSE ("值(信号)")
            # "设置"
            n853 = event-data() -> ()  [unwired: 1 in, 6 out]
          }
          event Panel Resize {
            # "允许全屏窗口"
            # "允许纵向调整"
            n854 = event-data() -> ("VIRef"=w1361:refnum<vi>, "NewBnds"=w1360:T30)  [unwired: 1 in, 6 out]
            n855 = disable-structure shown="禁用" {
              disable-tunnel: w1361 -> [w1366 _]
              disable-tunnel: w1360 -> [w1365 _]
              frame Disabled {
                n856 = Bundle By Name(cluster=w1365, "Left"="Left", "Right"="Right") -> (w1362:T30)
                n857 = property class="VI"(reference=w1366, "Front Panel.PanelBounds"=w1362) -> ()  [unwired: 1 in, 2 out]
              }
              frame Enabled {
              }
            }
          }
        }
      }
      n858 = local read "定时循环结构名称"() -> (w147:string)
      n859 = node-c288(w147) -> (w149:T19)  [unwired: 9 in]
      n860 = timed-loop {
        timing: w149 -> [_]
        timing-out: [_] -> w148
        i -> [w182]
        stop <- _ stop-if-true
        w181 = 5  # 滚动间隔
        # "周期性，从“通信单元”收集探头信息"
        n861 = node-c288() -> ()  [unwired: 1 in, 3 out]
        n862 = Quotient & Remainder(x=w182, y=w181) -> (x-y*floor(x/y)=w180:i32)  [unwired: 1 out]
        n863 = stacked-sequence {
          seq-local: [w202 _] -> [_ w213]
          frame #0 {
            w203 = T3 {"探头地址与信息"={"网络地址"="", "名称"="", "备注"="", "累积剂量"=0.0, "累积限值"=0.0, "硬件剂量率限值"=enum."一级限值", "剂量率限值1"=0.0, "剂量率限值2"=0.0, "报警方式"=enum."常报警"}, "测量值"={"时间"=timestamp(3554955153.6246996 s since 1904-01-01), "数值"=0.0}, "限值"={"限值1"=0.0, "限值2"=0.0, "探头限值"=enum."一级限值"}, "探头状态"=enum."正常", "累积记录"={"起始时间"=timestamp(0 s since 1904-01-01), "结束时间"=timestamp(0 s since 1904-01-01), "累积剂量"=0.0}, "报警方式"={"报警方式"=enum."常报警", "延迟计时"=0, "报警中？"=FALSE}}  # 探头属性
            # "收集探头属性，并以“信号”形式赋值，供监测窗口事件捕捉"
            n864 = for "For循环" {
              tunnel: "通信单元-探头属性引用[]" -> [w212] mode=indexing
              tunnel: w203 -> [w210]
              tunnel: [w209] -> w202 mode=indexing if=w205
              # "从“通信单元”获取属性值"
              n865 = property class="Ctl"(reference=w212) -> (error out=w208:errorcluster, "Value"=w211:variant)  [unwired: 1 in, 1 out]
              n866 = Variant To Data(error in=w208, type=w210, Variant=w211) -> (data=w209:T3, error out=w207:errorcluster)
              n867 = Unbundle By Name(w207) -> ("status"=w206:bool)
              n868 = Not "无错误？"(x=w206) -> (.not. x?=w205:bool)
            }
            n869 = Array Size(array=w202) -> (size(s)=w201:i32)
            n870 = property on="探头属性数组" class="Arr (严格)"("Val(Sgnl)"=w202) -> ()  [unwired: 2 in, 2 out]
            n871 = local write "探头数"(w201) -> ()
          }
          frame #1 {
            # "更新实时列表"
            n872 = case shown="假" "监测模式？" {
              tunnel: w213 -> [w216 w223]
              frame False {
                # "当前为列表窗口"
                n873 = case shown="假" "暂停更新？" {
                  tunnel: w216 -> [w219 _]
                  frame False {
                    # "更新"
                    n874 = control-ref of="实时数据列表"() -> (w218:refnum<vi>)
                    n875 = call "整合-测量信息至列表框-网络版.vi"("MCListbox引用句柄"=w218, "探头属性数组"=w219) -> ("测量状态"=w217:T2)  [unwired: 9 in]
                    n876 = property on="测量状态" class="Enum (严格)"("Val(Sgnl)"=w217) -> ()  [unwired: 2 in, 2 out]
                  }
                  frame True {
                    # "设置过程中，不更新"
                  }
                }
              }
              frame True {
                # "当前为探头模块窗口，不更新列表"
                n877 = for {
                  workers-P: _ -> [_]
                  tunnel: w223 -> [w230] mode=indexing
                  tunnel: [w229] -> w222 mode=indexing
                  # "构建侧脸状态数组"
                  n878 = Unbundle By Name(w230) -> ("探头状态"=w229:T9)
                }
                n879 = Array Max & Min(array=w222) -> (max value=w221:T9)  [unwired: 3 out]
                n880 = case shown="\"正常\", 默认" w221 {
                  tunnel: [测量状态."正常" 测量状态."一级报警" 测量状态."二级报警" 测量状态."累积报警" 测量状态."有掉线"] -> w220
                  frame "正常", Default {
                  }
                  frame "一级报警" {
                  }
                  frame "二级报警" {
                  }
                  frame "累积报警" {
                  }
                  frame "离线" {
                  }
                }
                n881 = property on="测量状态" class="Enum (严格)"("Val(Sgnl)"=w220) -> ()  [unwired: 2 in, 2 out]
              }
            }
          }
        }
        n882 = Equal To 0?(x=w180) -> (x = 0?=w179:bool)
        n883 = case shown="真" w179 {
          frame False {
          }
          frame True {
            w192 = 0 ("下限")
            w194 = 0 ("下限")
            # "滚动提示"
            n884 = Increment(x="设备列表提示索引") -> (x+1=w195:i32)
            n885 = Array Size(array="设备列表提示") -> (size(s)=w197:i32)
            n886 = Decrement(x=w197) -> (x-1=w184:i32)
            n887 = In Range and Coerce(upper limit=w184, x=w195, lower limit=w194) -> (In Range?=w196:bool)  [unwired: 1 out]
            n888 = Index Array(array="设备列表提示", index="设备列表提示索引") -> (element=→"设备列表操作提示":string)
            n889 = Select(t=w195, s=w196, f=w194) -> (s? t:f=w193:i32)
            n890 = local write "设备列表提示索引"(w193) -> ()
            n891 = Increment(x="报警列表提示索引") -> (x+1=w191:i32)
            n892 = Array Size(array="报警列表提示") -> (size(s)=w189:i32)
            n893 = Decrement(x=w189) -> (x-1=w183:i32)
            n894 = In Range and Coerce(upper limit=w183, x=w191, lower limit=w192) -> (In Range?=w190:bool)  [unwired: 1 out]
            n895 = Index Array(array="报警列表提示", index="报警列表提示索引") -> (element=→"报警列表操作提示":string)
            n896 = Select(t=w191, s=w190, f=w192) -> (s? t:f=w185:i32)
            n897 = local write "报警列表提示索引"(w185) -> ()
          }
        }
        n898 = node-c288() -> ()  [unwired: 1 in, 1 out]
      }
      n899 = node-c288(w148) -> ()  [unwired: 1 out]
      n900 = while {
        tunnel: "蜂鸣音效" -> [w154]
        tunnel: [w150] -> w146
        stop <- w155 stop-if-true
        # "报警声音播放"
        n901 = case shown="\"累积报警\"" "测量状态" {
          tunnel: [FALSE ("T") w159 w161 w162 w170] -> w151
          tunnel: [u32 500 ("等待时间（毫秒）") u32 500 ("等待时间（毫秒）") u32 0 ("等待时间（毫秒）") u32 500 ("等待时间（毫秒）") u32 500 ("等待时间（毫秒）")] -> w152
          frame "正常", Default {
            # "不报警"
          }
          frame "一级报警" {
            w159 = TRUE  # T
            # "间隔 0.5 s"
          }
          frame "二级报警" {
            w161 = TRUE  # T
            # "无间隔"
          }
          frame "累积报警" {
            # "禁用蜂鸣提示"
            n902 = disable-structure shown="启用" {
              disable-tunnel: [w164 _] -> w162
              frame Disabled {
                w167 = 0 ("y")
                w169 = 2  # 1s
                n903 = feedback #1(w167) -> (w165:i32)
                n904 = Greater Or Equal?(x=w165, y=w169) -> (x >= y?=w164:bool)
                n905 = Select(t=w167, s=w164, f=w165) -> (s? t:f=w168:i32)
                n906 = Increment(x=w168) -> (x+1=w166:i32)
                n907 = feedback-in #1(w166) -> ()
              }
              frame Enabled {
              }
            }
          }
          frame "有掉线" {
            w173 = 0 ("y")
            w175 = 6  # 3s
            # "间隔 3 s"
            n908 = feedback #2(w173) -> (w171:i32)
            n909 = Greater Or Equal?(x=w171, y=w175) -> (x >= y?=w170:bool)
            n910 = Select(t=w173, s=w170, f=w171) -> (s? t:f=w174:i32)
            n911 = Increment(x=w174) -> (x+1=w172:i32)
            n912 = feedback-in #2(w172) -> ()
          }
        }
        n913 = Wait (ms)(milliseconds to wait=w152) -> ()  [unwired: 1 out]
        n914 = case shown="真" w151 {
          tunnel: w154 -> [_ w178]
          tunnel: [_ w177] -> w150
          frame False {
          }
          frame True {
            n915 = call "播放波形"("Data"=w178) -> ("error out"=w177:errorcluster)  [unwired: 18 in]
          }
        }
        n916 = local read "停止"() -> (w155:bool)
      }
      n917 = call <vilib>:"Clear Errors.vi"("error in (no error)"=w146) -> ()  [unwired: 5 in, 2 out]
    }
  }
